vi "WHD_VEten_0.1_Pruebas.vi"() -> ()   [LabVIEW 2015]
uses:
  <vilib>/NI_Real-Time Target Support.lvlib
  <vilib>/rvi/interface/nirviReadWriteControl/nirviReadWriteControl.xnode
  <vilib>/rvi/interface/nirviMethod/nirviMethod.xnode
  <vilib>/rvi/interface/nirviOpenFPGA/nirviOpenFPGA.xnode
  <vilib>/rvi/interface/nirviCloseFPGA/nirviCloseFPGA.xnode
  <vilib>/real-time/NI_Real-Time Libraries.lvlib
  <vilib>/userdefined/High Color/nirio_resource_hc.ctl
  <vilib>/Utility/file.llb/Write To Spreadsheet File (string).vi
  AURA_Wheel/Json2Labv.lvlib
  AURA_Wheel/AuraWheelAPI/AuraWheel.lvlib
  <vilib>/LabVIEW Targets/FPGA/cRIO/shared/nicrio_ModuleControls/nicrio_cRIO-9234_DataRatesRing2.ctl
  FPGA Bitfiles/W&RDEuskotren_FPGATarget_FPGA8aws2_55B1237B.lvbitx
  <vilib>/real-time/rtutility.llb/RT Restart Target (Self).vi
  <vilib>/FPGAPlugInAG/cRIO-9113/niLvFpga_Open_cRIO-9113.vi
  <vilib>/FPGAPlugInAG/cRIO-9113/niLvFpga_Run_cRIO-9113.vi
  NiFpgaLv.dll
  <vilib>/Utility/error.llb/Error Cluster From Error Code.vi
  <vilib>/rvi/errors/niLvFpgaAdjustHostInterfaceError.vi
  <vilib>/FPGAPlugInAG/cRIO-9113/niLvFpga_ConfigureFifo_cRIO-9113.vi
  <vilib>/rvi/errors/niLvFpgaMergeErrorWithErrorCode.vi
  <vilib>/FPGAPlugInAG/cRIO-9113/niLvFpga_StartFifo_cRIO-9113.vi
  <vilib>/FPGAPlugInAG/cRIO-9113/niLvFpga_ReadFifo_cRIO-9113.vi
  <vilib>/FPGAPlugInAG/cRIO-9113/niLvFpga_StopFifo_cRIO-9113.vi
  <vilib>/FPGAPlugInAG/cRIO-9113/niLvFpga_Reset_cRIO-9113.vi
  <vilib>/FPGAPlugInAG/cRIO-9113/niLvFpga_Close_cRIO-9113.vi
  <vilib>/Utility/file.llb/Write Delimited Spreadsheet (string).vi
  <vilib>/RTwatchdog.llb/Watchdog expiration actions.ctl
panel:
  out "TAGs_AURAwheel":string[][](array[string])
  out "Plataformas?":bool
  out "Ejes_convoy":i32
  out "Nº Ejes":i32[](array[numeric])
  out "Nº UTs":i32
  out "it-read-LR6":i32[](array[numeric])
  out "it-LR6":i32
  out "RFID_LR6_Error":errorcluster
  out "TAGs HEX":string[](array[string])
  out "TAGs LR6":string[](array[string])
  in  "TAGs HEX 2":string[](array[string])
  out "Series_flota":string[](array[string])
  out "Tabla_flota":string[][](array[string])
  out "Puntos medios de las ventanas":dbl[][](array[numeric])
  in  "User":string
  in  "Índice de los archivos seleccionados":i32
  in  "Array":path[][](array[path])=[[path "c:/Trenes_prueba/0207_2013-09-24_19-09-42_0.bin", path "c:/Trenes_prueba/0096_2013-10-30_18-13-14_0.bin", path "c:/Trenes_prueba/0001_2013-06-05_13-06-23_0.bin"], [path "c:/Trenes_prueba/0207_2013-09-24_19-09-42_1.bin", path "c:/Trenes_prueba/0096_2013-10-30_18-13-14_1.bin", path "c:/Trenes_prueba/0001_2013-06-05_13-06-23_1.bin"], [path "c:/Trenes_prueba/0207_2013-09-24_19-09-42_2.bin", path "c:/Trenes_prueba/0096_2013-10-30_18-13-14_2.bin", path "c:/Trenes_prueba/0001_2013-06-05_13-06-23_2.bin"], [path "c:/Trenes_prueba/0207_2013-09-24_19-09-42_3.bin", path "c:/Trenes_prueba/0096_2013-10-30_18-13-14_3.bin", path "c:/Trenes_prueba/0001_2013-06-05_13-06-23_3.bin"], [path "c:/Trenes_prueba/0207_2013-09-24_19-09-42_4.bin", path "c:/Trenes_prueba/0096_2013-10-30_18-13-14_4.bin", path "c:/Trenes_prueba/0001_2013-06-05_13-06-23_4.bin"], [path "c:/Trenes_prueba/0207_2013-09-24_19-09-42_5.bin", path "c:/Trenes_prueba/0096_2013-10-30_18-13-14_5.bin", path "c:/Trenes_prueba/0001_2013-06-05_13-06-23_5.bin"], [path "c:/Trenes_prueba/0207_2013-09-24_19-09-42_6.bin", path "c:/Trenes_prueba/0096_2013-10-30_18-13-14_6.bin", path "c:/Trenes_prueba/0001_2013-06-05_13-06-23_6.bin"], [path "c:/Trenes_prueba/0207_2013-09-24_19-09-42_7.bin", path "c:/Trenes_prueba/0096_2013-10-30_18-13-14_7.bin", path "c:/Trenes_prueba/0001_2013-06-05_13-06-23_7.bin"], [path "c:/Trenes_prueba/0207_2013-09-24_19-09-42_8.bin", path "c:/Trenes_prueba/0096_2013-10-30_18-13-14_8.bin", path "c:/Trenes_prueba/0001_2013-06-05_13-06-23_8.bin"]]
  out "configuration file path":path=path "c:/Parametros.cfg"
  in  "IP synchr":string
  in  "Canal ccero?":bool
  in  "Digital?":bool=TRUE
  out "Numeric 3":i32
  out "data":cluster{"status":string}
  out "confRFID":path=path "c:/RFID/TAGS.csv"
  out "TAGS leidos":path=path "c:/RFID/TAGS.csv"
  in  "Use Aura?":bool
  in  "Parametros AuraWheel":string[](array[string])
  in  "Parámetros acelerómetros":dbl[](array[numeric])
  in  "Number of Samples":u32=2000
  in  "x*y":dbl[](array[numeric])=array[252000 elements]
  out "RFID_Error 2":errorcluster
  in  "milliseconds to wait":u32=180000
  in  "Adquirir continuado":bool
  in  "Tiempo de adquisicion":dbl=10.0
  in  "Adquirir":bool
  in  "Señal digital?":bool=TRUE
  out "Inductivo OK?":bool=TRUE
  out "Acelerómetros OK?":bool[](array[boolean])
  out "Fin":bool
  out "Contador":i32=1
  in  "expiration actions":T1={"reset"=TRUE, "occurrence"=FALSE, "trigger protocol"=enum."active high", "trigger line"=enum."none", "disable watchdog on VI exit"=TRUE}
  out "Path TEST":path=path "c:/TEST"
  out "Fallo fotocelula":bool
  out "Path_Borrar":path=path "c:/Trenes"
  out "Longitud de la unidad":dbl
  out "Bucle Espera":i32
  out "Aviso no detección":string
  out "Time to Acquire Block (ms)":i32
  out "Distancia de acelerómetros":dbl[](array[numeric])
  out "Block Size":u32
  out "Distancias generales":dbl[](array[numeric])
  in  "Reset del controlador":bool
  in  "Configuración":bool
  in  "Parar la aplicación":bool
  out "Acel 4":bool=TRUE
  out "Acel 3":bool=TRUE
  out "Acel 2":bool=TRUE
  out "Acel 1":bool=TRUE
  out "RFID":bool=TRUE
  out "date/time string":string
  out "Obstruido?":bool
  out "Tiempo":dbl
  out "Inicio pasada":timestamp
  out "Ultimo TEST":timestamp
  out "Fuente":bool=TRUE
  out "Estado":string
  in  "Number of Channels":u32=9
  out "RFID_ID":refnum<k5>
  out "DC OK":string
  out "Aviso temperatura":string
  in  "Tab Control":T2(tab)=enum."Parámetros"
  out "V (m/s)":dbl
  out "Temperatura (ºC)":dbl
  out "Max RMS Ruedas":dbl[][](array[numeric])
  in  "Hora de borrado":string
  out "result":bool
  out "TAGs":string[](array[string])
  out "Nombre de archivo":path[](array[path])
  out "Tiempo de paso (s)":dbl
  out "Tiempo extra de adquisición (s)":dbl
  out "Número de ejes detectados":i32
  out "Buffer Underflow":bool
  out "Buffer Overflow":bool
  out "Disco Duro Disponible (bytes)":i64
  out "created path":path
  out "Fallo sensores":string
  out "T fuera rango":bool
  in  "Frecuencia de muestreo (Hz)":dbl=25600.0
  in  "Escaneos de la FIFO por canal":u32=1000
  in  "Tiempo extra al detector de paso (s)":dbl=1.0
  in  "Filtro digital (ms)":u16=13
  in  "dt RMS":dbl=256.0
  in  "Time":T3 {"Segundo" min=0 max=60; "Minuto" min=0 max=60; "Hora" min=0 max=24}
  in  "Cambiar hora":bool
  in  "Date":T4={"Mes   "=1, "Día         "=1, "Año "=2010} {"Año" min=1900 max=3000 step=1; "Día" min=1 max=31 step=1; "Mes" min=1 max=12 step=1}
  in  "Cambiar Fecha":bool
  in  "Frecuencia de muestreo y módulo CRIO":T5=2 items=["51.200 kS/s (NI 9234)"=1, "25.600 kS/s (NI 9234)"=2, "17.067 kS/s (NI 9234)"=3, "12.800 kS/s (NI 9234)"=4, "10.240 kS/s (NI 9234)"=5, "8.533 kS/s (NI 9234)"=6, "7.314 kS/s (NI 9234)"=7, "6.400 kS/s (NI 9234)"=8, "5.689 kS/s (NI 9234)"=9, "5.120 kS/s (NI 9234)"=10, "4.654 kS/s (NI 9234)"=11, "4.267 kS/s (NI 9234)"=12, "3.938 kS/s (NI 9234)"=13, "3.657 kS/s (NI 9234)"=14, "3.413 kS/s (NI 9234)"=15, "3.200 kS/s (NI 9234)"=16, "3.012 kS/s (NI 9234)"=17, "2.845 kS/s (NI 9234)"=18, "2.695 kS/s (NI 9234)"=19, "2.560 kS/s (NI 9234)"=20, "2.438 kS/s (NI 9234)"=21, "2.328 kS/s (NI 9234)"=22, "2.226 kS/s (NI 9234)"=23, "2.133 kS/s (NI 9234)"=24, "2.048 kS/s (NI 9234)"=25, "1.969 kS/s (NI 9234)"=26, "1.896 kS/s (NI 9234)"=27, "1.829 kS/s (NI 9234)"=28, "1.765 kS/s (NI 9234)"=29, "1.707 kS/s (NI 9234)"=30, "1.652 kS/s (NI 9234)"=31]
  in  "Puerto RFID":u16=2189
  in  "IP RFID":string="192.168.106.99"
  in  "Offset_rueda":fxp<+/-,24,-4>=0.004999998956918716 format="%.27g"
  in  "Count(mSec)":u32=2
  in  "LR6 IP address":string="192.168.106.94"
  in  "Port LR6":u16=2001
  in  "Pruebas RFID 2":bool
  in  "Pruebas RFID 1":bool
  in  "Descargar":bool
  out "Parámetros":bool=TRUE
  out "Distacias y medidas de dispositivos":bool=TRUE
  out "RFID_Error":errorcluster
  out "error FPGA":errorcluster
  out "error manipulacion archivos":errorcluster
  out "Unidades y ejes":bool=TRUE
  out "RFID":bool=TRUE
  out "error AURA":errorcluster
  out "Response headers":string
  # "Funciona?"
  # "Inductivo"
  # "A4"
  # "A3"
  # "A1"
  # "A2"
  # "WRD_MEX\nWRD_ZAR"
  # "0 tagMexInit\n1 tagMexFin\n\n0 tag1\n1 tag2"
  # "Última detección de unidad"
  # "Error!!"
  # "Estado de la memoria"
  # "Espera"
  # "Adquisicion"
  # "Adquisicion"
  # "Procesado"
  # "Procesado"
  # "Procesado"
  # "Procesado"
  # "Procesado"
  # "Parámetros de muestreo"
  # "Parámetros de adquisición"
  # "Parámetros de procesado"
  # "Cambio Fecha y Hora"
  # "Descarga de planos y TEST"
  # "NO"
  # "SI"
  # "Descarga archivos binarios de adquisición"
  # "NO"
  # "SI"
  # "Cargar datos de configuración"
  # "Errores!!"
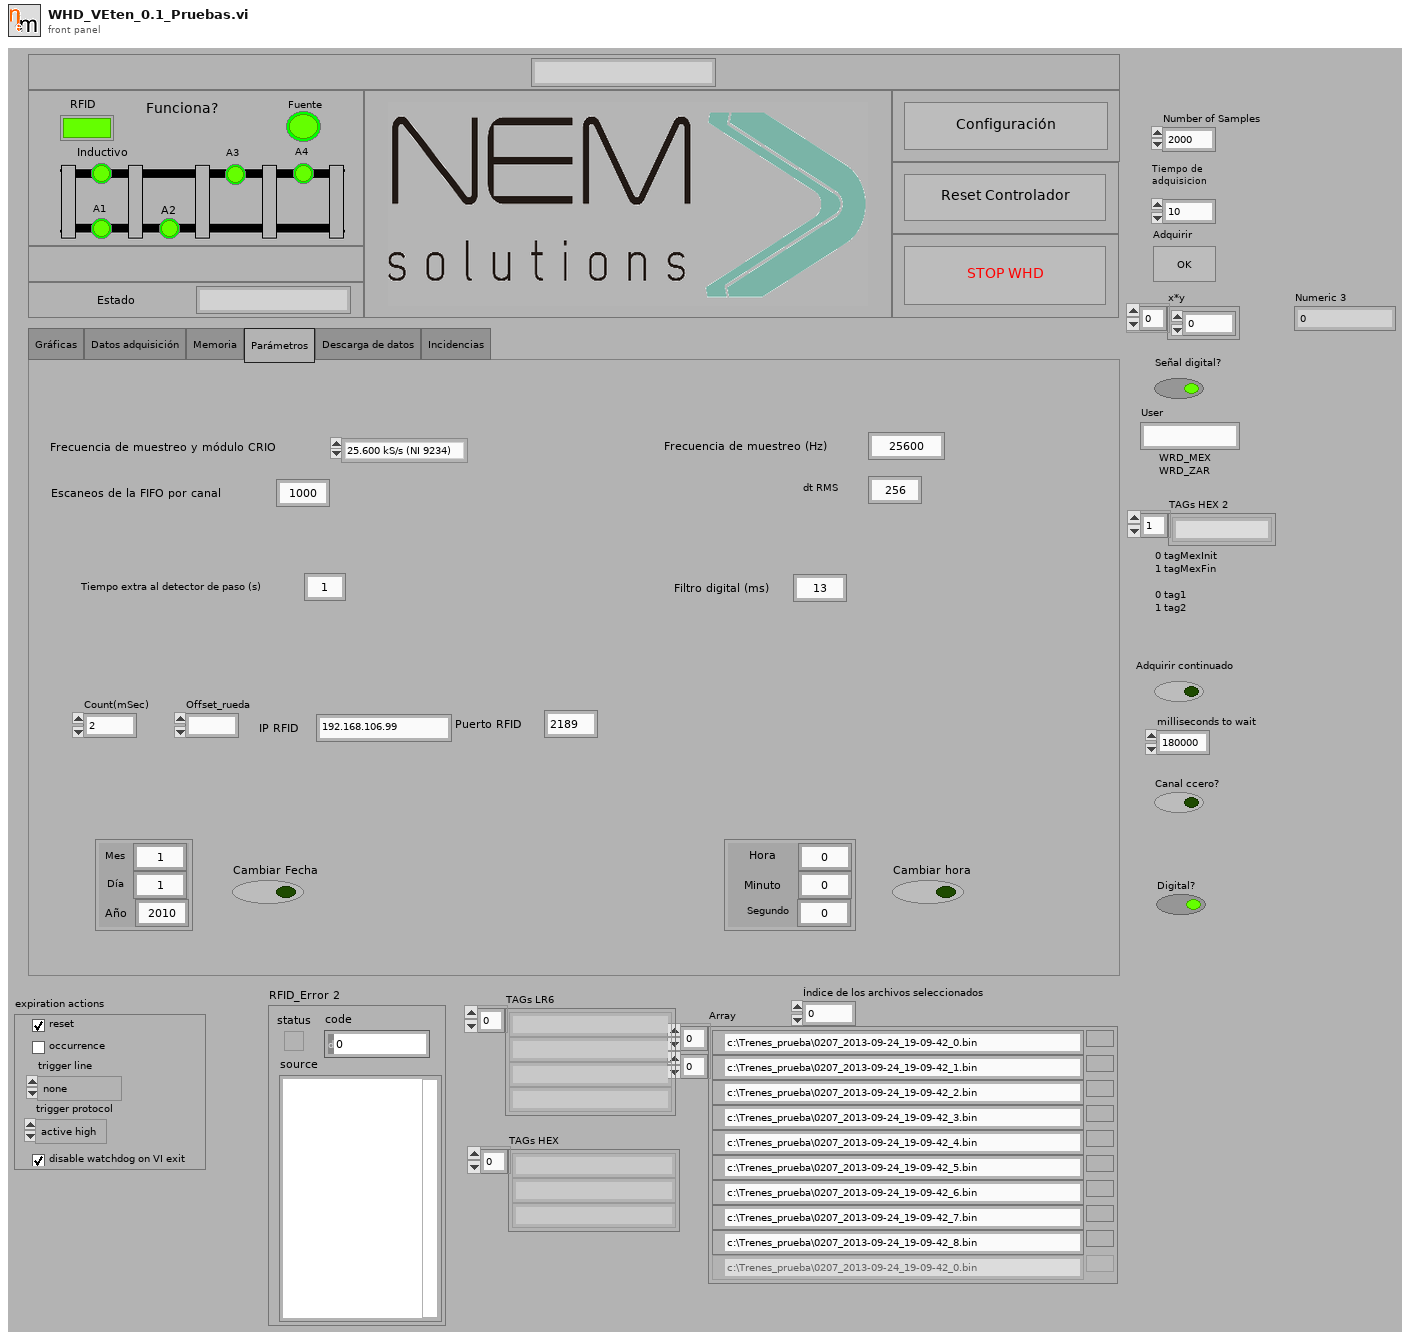
[diagram p1: front panel]
types:
  T1 = typedef "Watchdog expiration actions.ctl" = cluster{"reset":bool, "occurrence":bool, "trigger protocol":enum16{"active high", "active low", "open collector"}, "trigger line":enum16{"none", "line 0", "line 1", "line 2", "line 3", "line 4", "line 5", "line 6", "line 7", "SMB line 0"}, "disable watchdog on VI exit":bool}
  T2 = enum32{"Gráficas", "Datos adquisición", "Memoria", "Parámetros", "Descarga de datos", "Incidencias"}
  T3 = cluster{"Hora        ":i32, "Minuto     ":i32, "Segundo               ":i32}
  T4 = cluster{"Mes   ":i32, "Día         ":i32, "Año ":i32}
  T5 = typedef "nicrio_cRIO-9234_DataRatesRing2.ctl" = u8
  T6 = typedef "nirio_resource_hc.ctl" = tag
  T7 = enum16{"Standard", "Buffered", "CRLF", "Immediate"}
  T8 = enum16{"open", "replace", "create", "open or create", "replace or create", "replace or create with confirmation"}
  T9 = enum16{"big-endian, network order", "native, host order", "little-endian"}
  T10 = cluster{"error IO":errorcluster, bool[], u32[], string[], dbl[]}
  T11 = cluster{"g_ts":dbl, "p_sp":dbl, "p_tp":dbl, "p_tg":cluster{"tg_n":dbl, "tg_t":string}[], "p_ax":cluster{"ax_n":dbl, "ax_sp":dbl, "ax_wh":cluster{"wh_p":dbl, "wh_a1":dbl, "wh_a2":dbl, "wh_a3":dbl, "wh_a4":dbl}[]}[]}
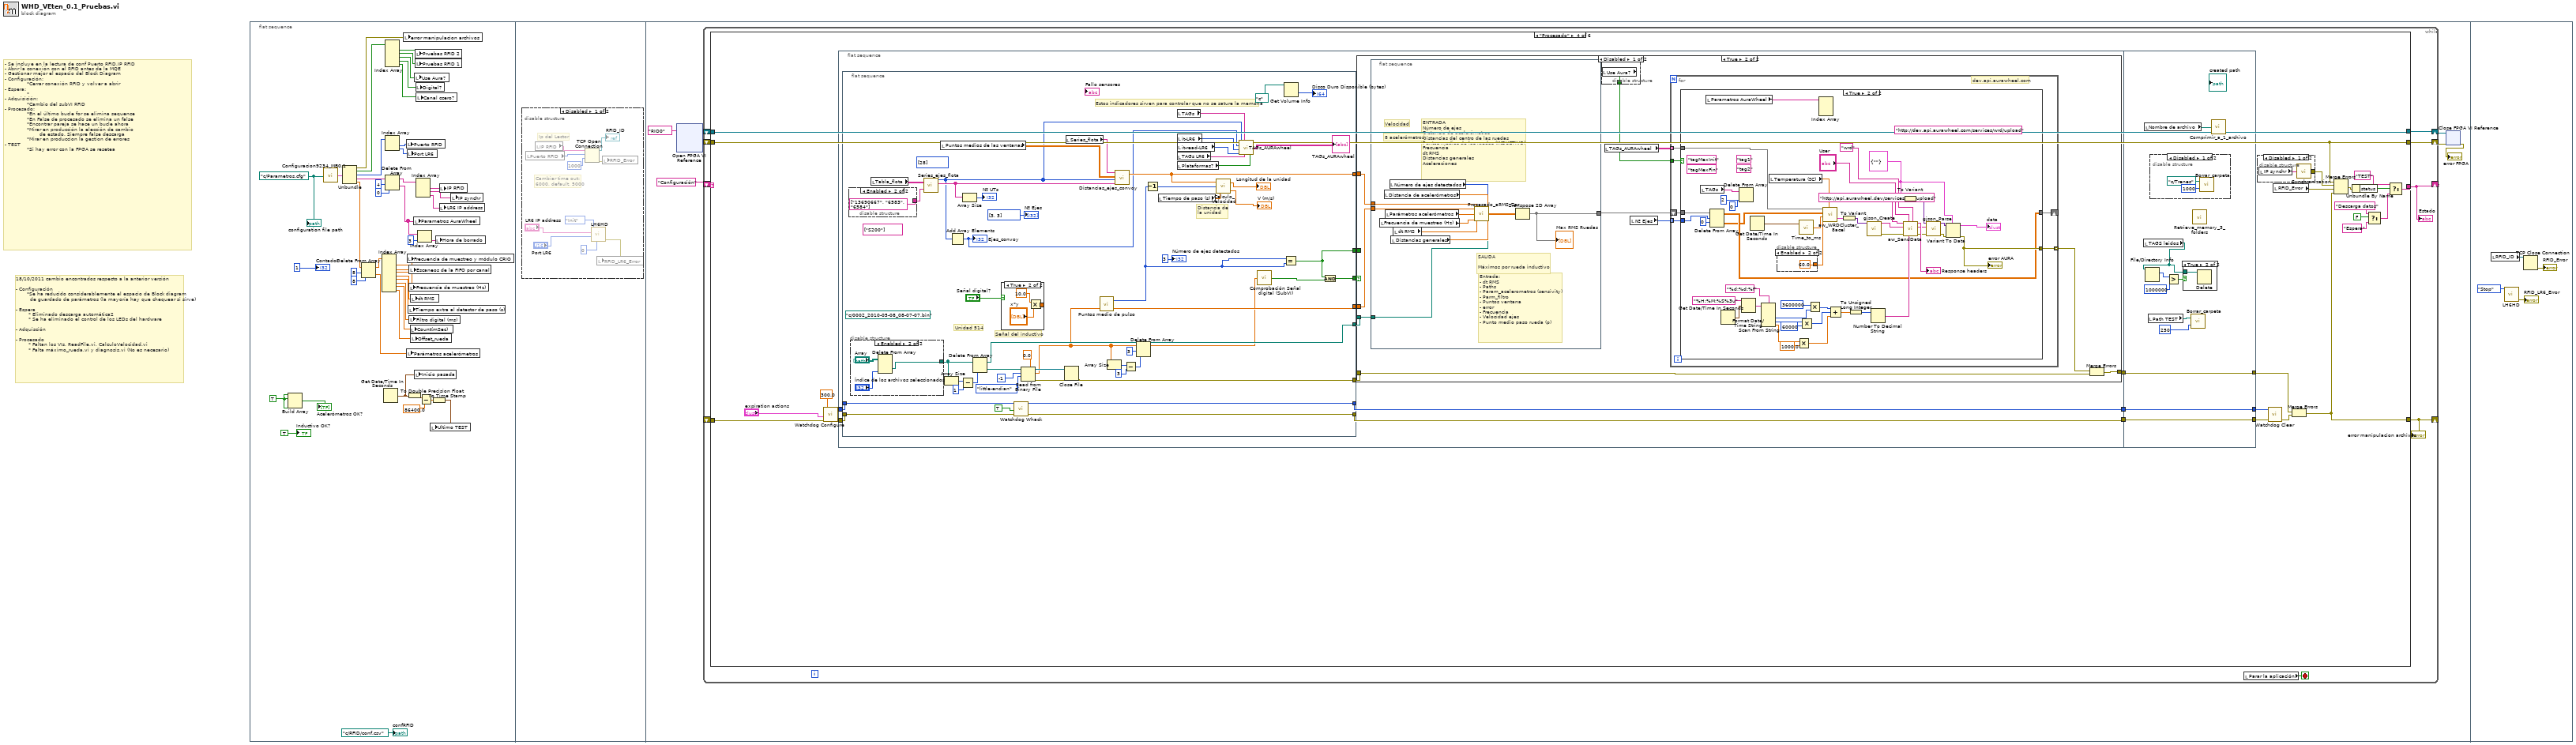
[diagram p0: block diagram]
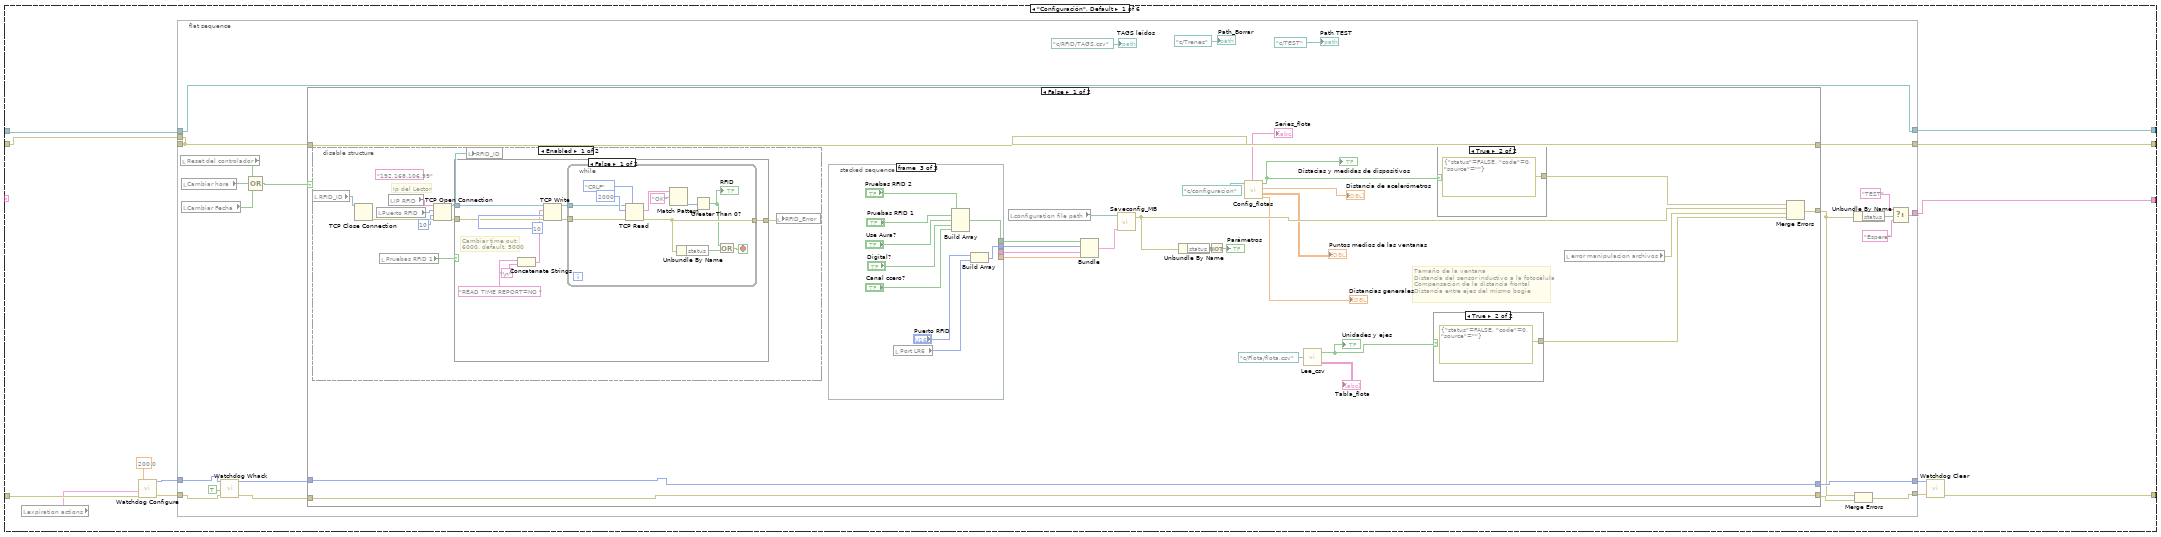
[diagram p3: hidden frame]
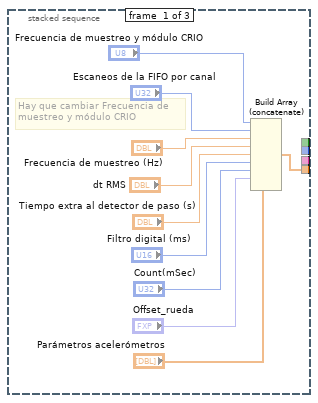
[diagram p4: hidden frame]
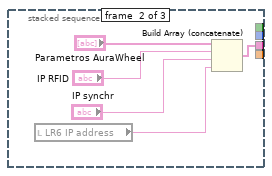
[diagram p5: hidden frame]
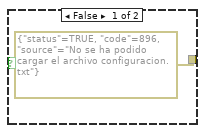
[diagram p6: hidden frame]
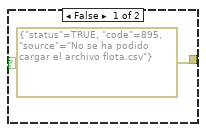
[diagram p7: hidden frame]
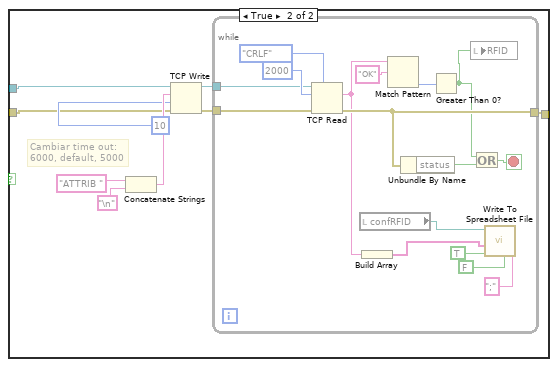
[diagram p8: hidden frame]
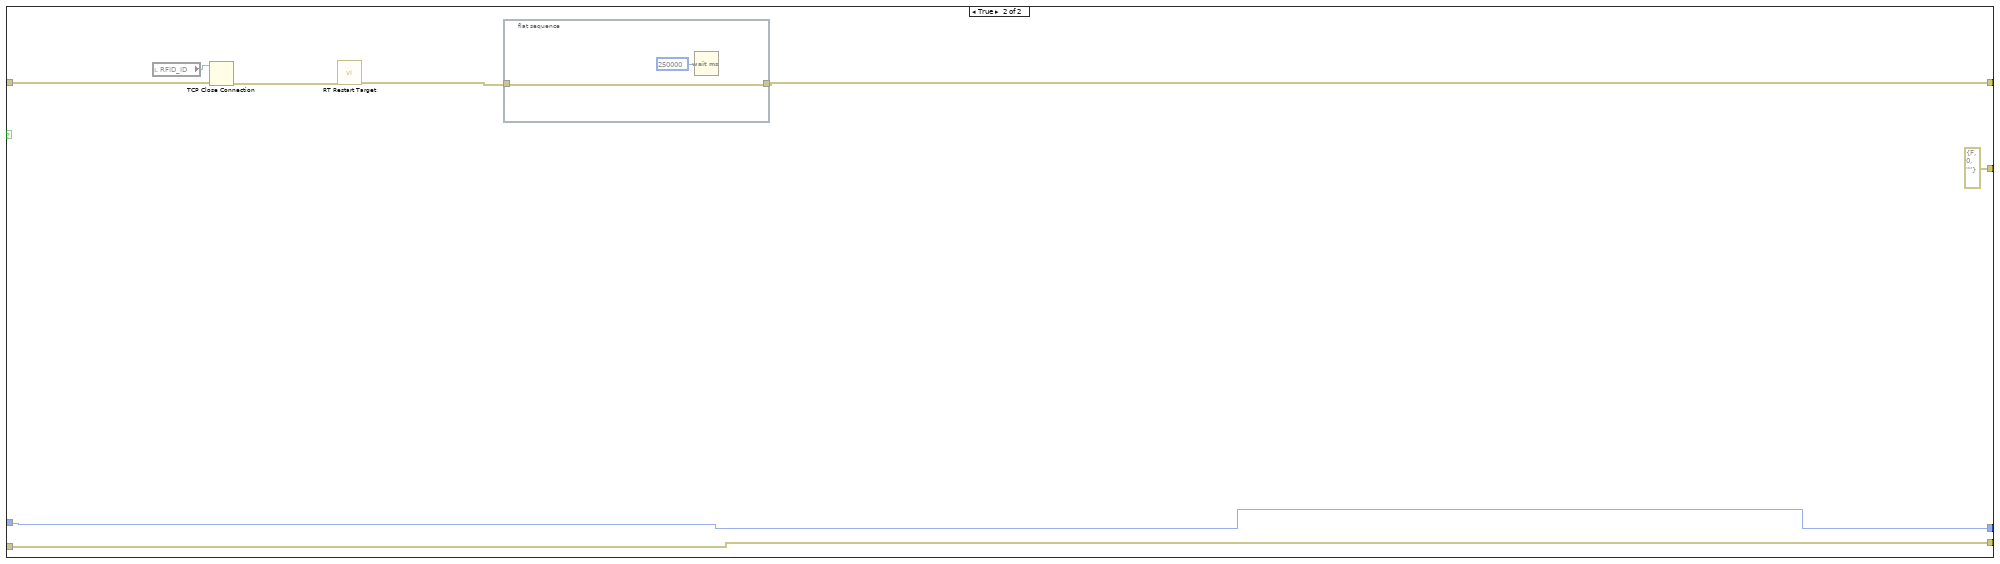
[diagram p10: hidden frame]
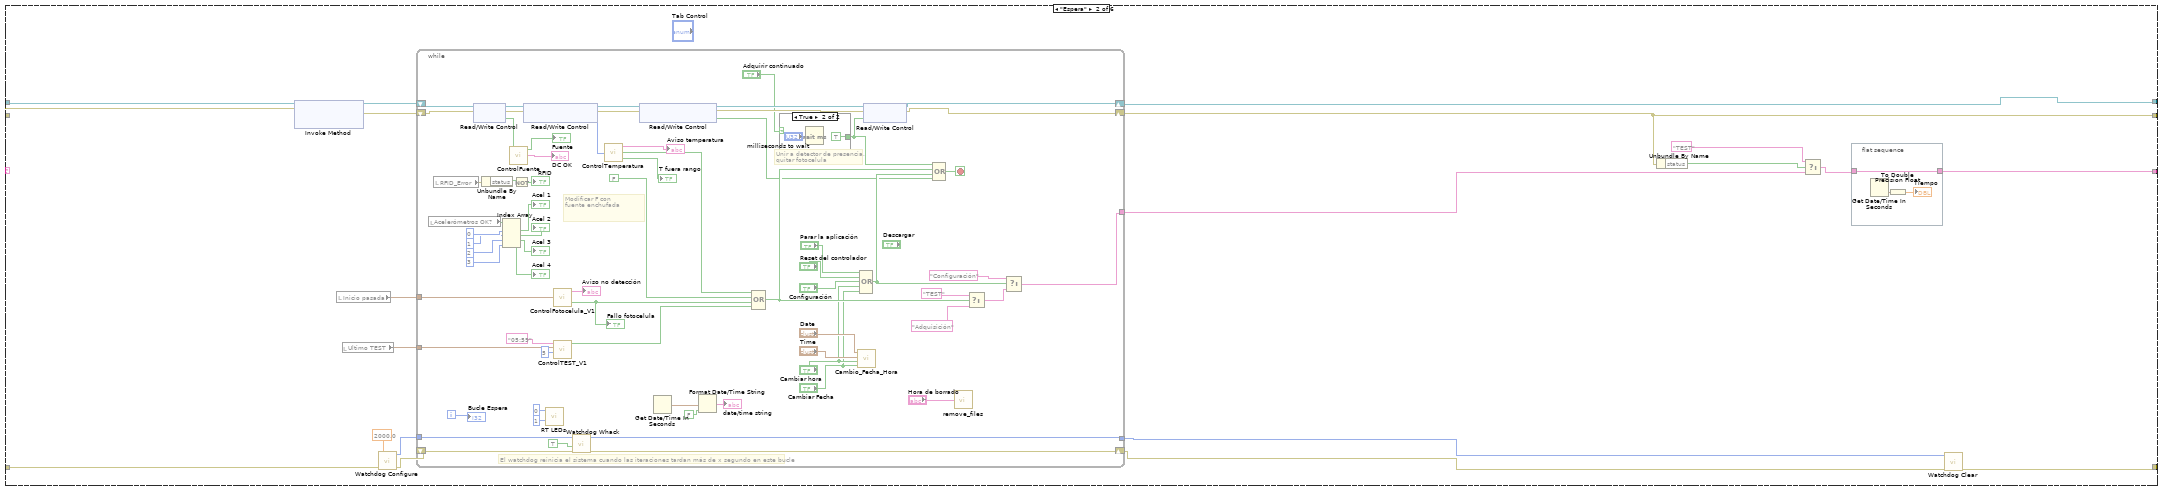
[diagram p11: hidden frame]
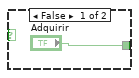
[diagram p12: hidden frame]
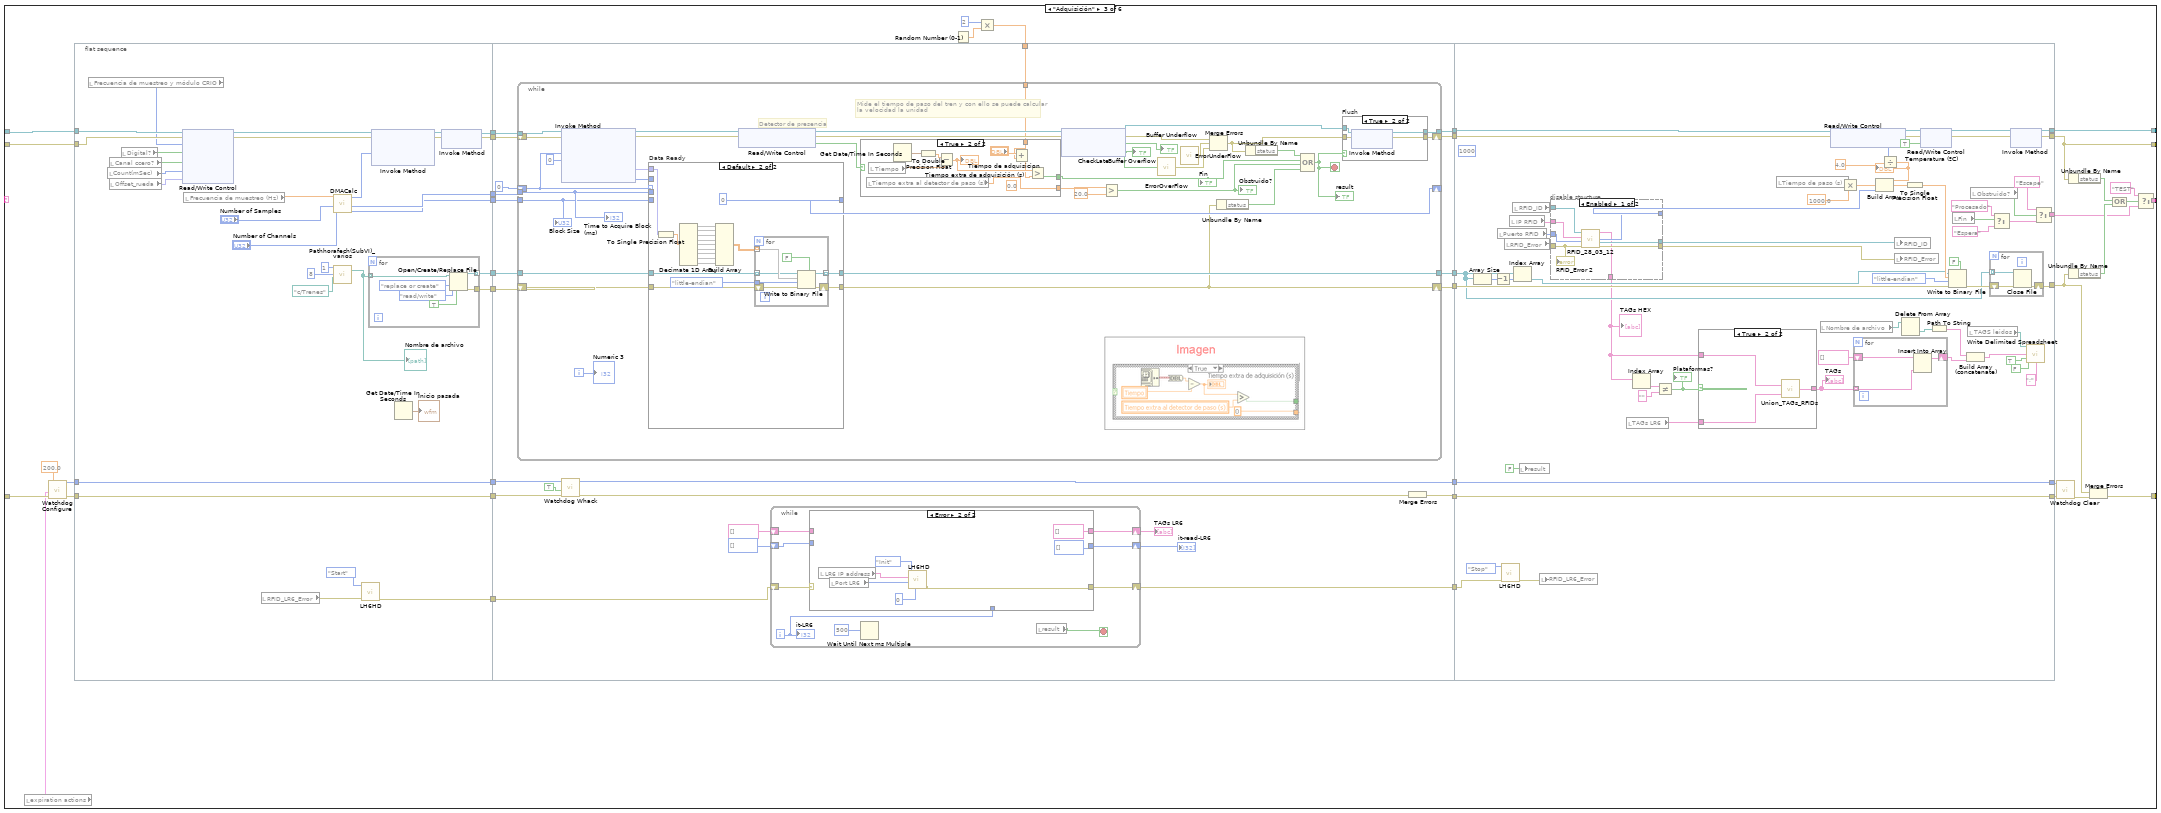
[diagram p13: hidden frame]
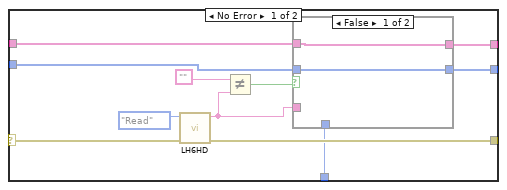
[diagram p14: hidden frame]
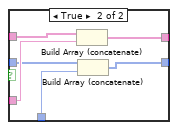
[diagram p15: hidden frame]
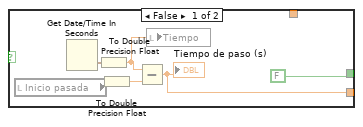
[diagram p16: hidden frame]
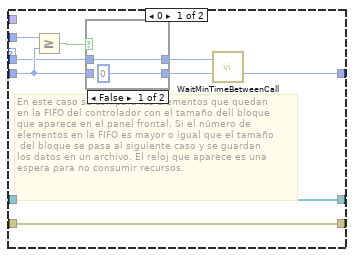
[diagram p17: hidden frame]
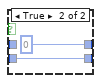
[diagram p18: hidden frame]
diagram:
  # "18/10/2011 cambio encontrados respecto a la anterior versión\n\n- Configuración\n       *Se ha reducido considerablemente el espacio de Block diagram\n         de guardado de parámetros (la mayoría hay que chequear si sirve)\n\n- Espera\n        * Eliminado descarga automática2\n        * Se ha eliminado el control de los LEDs del hardware\n       \n- Adquisción\n\n- Procesado\n        * Faltan los VIs, ReadFile.vi, CalculoVelocidad.vi\n        * Falta máximo_rueda.vi y diagnosis.vi (No es necesario)"
  # "- Se incluye en la lectura de conf Puerto RFID,IP RFID\n- Abrir la conexión con el RFID antes de la MQE\n- Gestionar mejor el espacio del Block Diagram\n- Configuración:\n              *Cerrar conexión RFID y volver a abrir\n- Espera:\n              *\n- Adquisición:\n              *Cambio del subVI RFID\n- Procesado:\n              *En el último bucle for se elimina sequence\n              *En False de procesado se elimina un false\n              *Encontrar pareja se hace un bucle ahora\n              *Mirar en producción la elección de cambio\n                      de estado. Siempre false descarga \n              *Mirar en produccion la gestion de errores\n- TEST\n              *Si hay error con la FPGA se resetea"
  n1 = flat-sequence {
    frame #0 {
      w29 = TRUE
      w25 = path "c:/Parametros.cfg" ("configuration file path")
      n2 = Build Array(w29, w29, w29, w29) -> (→"Acelerómetros OK?":bool[])
      n3 = call "Configuracion9234_MB0.1.vi"("configuration file path"=w25) -> ("output cluster"=w24:T10)
      n4 = Unbundle(w24) -> ("error IO"=w32:errorcluster, w31:bool[], w30:u32[], w16:string[], w22:dbl[])
      n5 = Delete From Array(array=w22, length=8, index=8) -> (deleted portion=w18:dbl[], array with subset deleted=w21:dbl[])
      n6 = Index Array(array=w21) -> (element #1=w40:dbl, element #2=w39:dbl, element #3=w38:dbl, element #4=w37:dbl, element #5=w36:dbl, element #6=w35:dbl, element #7=w8:dbl, element #8=w7:dbl)  [unwired: 8 in]
      n7 = Get Date/Time In Seconds() -> (seconds since 1Jan1904=w42:timestamp)
      n8 = Index Array(array=w31) -> (element #1=w34:bool, element #2=w33:bool, element #3=w17:bool, element #4=w4:bool, element #5=w9:bool)  [unwired: 5 in]
      n9 = Index Array(array=w30) -> (element #1=w23:u32, element #2=w1:u32)  [unwired: 2 in]
      n10 = Delete From Array(array=w16, length=4, index=0) -> (deleted portion=w5:string[], array with subset deleted=w15:string[])
      n11 = local write "error manipulacion archivos"(w32) -> ()
      n12 = local write "Puerto RFID"(w23) -> ()
      n13 = local write "Parámetros acelerómetros"(w18) -> ()
      n14 = local write "Port LR6"(w1) -> ()
      n15 = local write "Frecuencia de muestreo y módulo CRIO"(w40) -> ()
      n16 = To Double Precision Float(number=w42) -> (double precision float=w44:dbl)
      n17 = local write "Tiempo extra al detector de paso (s)"(w36) -> ()
      n18 = local write "Frecuencia de muestreo (Hz)"(w38) -> ()
      n19 = local write "Filtro digital (ms)"(w35) -> ()
      n20 = local write "Escaneos de la FIFO por canal"(w39) -> ()
      n21 = local write "Count(mSec)"(w8) -> ()
      n22 = local write "dt RMS"(w37) -> ()
      n23 = local write "Offset_rueda"(w7) -> ()
      n24 = local write "Parametros AuraWheel"(w5) -> ()
      n25 = local write "Inicio pasada"(w42) -> ()
      n26 = local write "Use Aura?"(w17) -> ()
      n27 = local write "Pruebas RFID 2"(w34) -> ()
      n28 = local write "Pruebas RFID 1"(w33) -> ()
      n29 = local write "Digital?"(w4) -> ()
      n30 = Index Array(array=w15) -> (element #1=w3:string, element #2=w6:string, element #3=w2:string)  [unwired: 3 in]
      n31 = local write "Canal ccero?"(w9) -> ()
      n32 = Index Array(array=w5, index=3) -> (element=w10:string)
      n33 = Subtract(x=w44, y=86400.0) -> (x-y=w43:dbl)
      n34 = To Time Stamp(1:w43) -> (0:w41:timestamp)
      n35 = local write "Ultimo TEST"(w41) -> ()
      n36 = local write "Hora de borrado"(w10) -> ()
      n37 = local write "IP RFID"(w3) -> ()
      n38 = local write "LR6 IP address"(w2) -> ()
      n39 = local write "IP synchr"(w6) -> ()
      "Contador" <- 1
      "Inductivo OK?" <- TRUE ("Inductivo OK?")
      "confRFID" <- path "c:/RFID/conf.csv" ("file path (use dialog)")
      "configuration file path" <- w25
    }
    frame #1 {
      n40 = disable-structure shown="Disabled" {
        frame Disabled {
          # "Cambiar time out:\n6000, default, 5000"
          # "Ip del Lector"
          n41 = local read "Puerto RFID"() -> (w52:u16)
          n42 = local read "IP RFID"() -> (w53:string)
          n43 = TCP Open Connection(address=w53, remote port or service name=w52, timeout ms (60000)=1000) -> (connection ID=→"RFID_ID":refnum<k5>, error out=w51:errorcluster)  [unwired: 1 in, 1 out]
          n44 = call "LH6HD.vi"("DeviceAddress"=u8 0, "Reader Port"="Port LR6", "IP Address"="LR6 IP address", "Action"=enum16{"Init", "Start", "Read", "Stop", "Exit"}."Init") -> ("error out"=w50:errorcluster)  [unwired: 6 in, 1 out]
          n45 = local write "RFID_LR6_Error"(w50) -> ()
          n46 = local write "RFID_Error"(w51) -> ()
        }
        frame Enabled {
        }
      }
    }
    frame #2 {
      n47 = xnode "Open FPGA VI Reference"("resource name"=T6 "RIO0") -> ("FPGA VI Reference Out"=w62:refnum<k20>, "error out"=w61:errorcluster)  [unwired: 1 in]
      n48 = while {
        shift-right: [w66] -> _
        shift-left: "Configuración" -> [w71]
        shift-right: [w64] -> w58
        shift-left: w62 -> [w70]
        shift-right: [w63] -> w57
        shift-left: w61 -> [w69]
        shift-right: [w68] -> _
        shift-left: _ -> [w67]
        stop <- w65 stop-if-true
        n49 = case shown="\"Procesado\"" w71 {
          tunnel: [w83 w228 w324 w638 w858 "TEST" ("t")] -> w66
          tunnel: [w82 w227 w345 w653 w856 w925] -> w64
          tunnel: [w84 w225 w346 w630 w847 w922] -> w63
          tunnel: w70 -> [w73 w234 w356 w653 w856 w924]
          tunnel: w69 -> [w72 w232 w355 w630 w855 w921]
          tunnel: [w75 w226 w341 w635 w854 w926] -> w68
          tunnel: w67 -> [w80 w242 w347 w651 w857 w926]
          frame "Configuración", Default {
            n50 = local read "expiration actions"() -> (w74:T1)
            n51 = call <vilib>:"Watchdog Configure.vi"("error in (no error)"=w80, "expiration actions"=w74, "timeout (1 sec)"=200.0) -> ("error out"=w79:errorcluster, "watchdogID"=w78:u64)  [unwired: 3 out]
            n52 = flat-sequence {
              tunnel: [w85] -> _
              tunnel: [w94] -> w84
              tunnel: [w106] -> w83
              tunnel: w73 -> [w95]
              tunnel: [w95] -> w82
              tunnel: w79 -> [w89]
              tunnel: w78 -> [w87]
              tunnel: [w93] -> w77
              tunnel: [w97] -> w76
              tunnel: w72 -> [w85]
              frame #0 {
                n53 = local read "Reset del controlador"() -> (w102:bool)
                n54 = local read "Cambiar hora"() -> (w101:bool)
                n55 = local read "Cambiar Fecha"() -> (w100:bool)
                n56 = call <vilib>:"Watchdog Whack.vi"("error in (no error)"=w89, "reset watchdog after expire? (F)"=TRUE, "watchdogID in"=w87) -> ("error out"=w88:errorcluster, "watchdogID out"=w86:u64)  [unwired: 3 out]
                n57 = Compound Arithmetic op=OR(w102, w101, w100) -> (w99:bool)
                n58 = case shown="False" w99 {
                  tunnel: w85 -> [w132 w220]
                  tunnel: [w132 w217] -> w94
                  tunnel: [w118 errorcluster {"status"=FALSE, "code"=0, "source"=""} ("error IO")] -> w92
                  tunnel: w86 -> [w117 w216]
                  tunnel: w88 -> [w116 w215]
                  tunnel: [w117 w216] -> w93
                  tunnel: [w116 w215] -> w91
                  frame False {
                    # "Tamaño de la ventana\nDistancia del sensor inductivo a la fotocélula\nCompensación de la distancia frontal\nDistancia entre ejes del mismo bogie"
                    n59 = disable-structure shown="Enabled" {
                      frame Enabled {
                        (unwired) "192.168.106.99" ("address")
                        # "Ip del Lector"
                        n60 = local read "RFID_ID"() -> (w168:refnum<k5>)
                        n61 = TCP Close Connection(connection ID=w168) -> (error out=w169:errorcluster)  [unwired: 2 in, 1 out]
                        n62 = local read "Puerto RFID"() -> (w166:u16)
                        n63 = local read "Pruebas RFID 1"() -> (w161:bool)
                        n64 = local read "IP RFID"() -> (w165:string)
                        n65 = TCP Open Connection(address=w165, remote port or service name=w166, timeout ms (60000)=10, error in (no error)=w169) -> (connection ID=w167:refnum<k5>, error out=w162:errorcluster)  [unwired: 1 out]
                        n66 = case shown="False" w161 {
                          tunnel: w167 -> [w178 w192]
                          tunnel: [w176 w190] -> w163
                          tunnel: w162 -> [w173 w191]
                          frame False {
                            # "Cambiar time out:\n6000, default, 5000"
                            n67 = Concatenate Strings("READ TIME REPORT=NO " ("data in"), "\n") -> (w170:string)
                            n68 = TCP Write(connection ID=w178, data in=w170, error in (no error)=w173, 9:10 ("timeout ms (25000)")) -> (connection ID out=w174:refnum<k5>, error out=w175:errorcluster)  [unwired: 1 out]
                            n69 = while {
                              tunnel: w175 -> [w187]
                              tunnel: w174 -> [w186]
                              tunnel: [w185] -> w176
                              stop <- w182 stop-if-true
                              n70 = TCP Read(connection ID=w186, bytes to read=2000, error in (no error)=w187, 7:T7."CRLF" ("mode (standard)")) -> (data out=w180:string, error out=w185:errorcluster)  [unwired: 1 in, 1 out]
                              n71 = Match Pattern(string=w180, regular expression="OK") -> (offset past match=w183:i32)  [unwired: 4 out]
                              n72 = Unbundle By Name(w185) -> ("status"=w181:bool)
                              n73 = Greater Than 0?(x=w183) -> (x > 0?=w179:bool)
                              "RFID" <- w179
                              n74 = Or(x=w179, y=w181) -> (x .or. y?=w182:bool)
                            }
                          }
                          frame True {
                            # "Cambiar time out:\n6000, default, 5000"
                            n75 = Concatenate Strings("ATTRIB " ("data in"), "\n") -> (w198:string)
                            n76 = TCP Write(connection ID=w192, data in=w198, error in (no error)=w191, 9:10 ("timeout ms (25000)")) -> (connection ID out=w195:refnum<k5>, error out=w194:errorcluster)  [unwired: 1 out]
                            n77 = while {
                              tunnel: w194 -> [w212]
                              tunnel: w195 -> [w211]
                              tunnel: [w210] -> w190
                              stop <- w207 stop-if-true
                              n78 = TCP Read(connection ID=w211, bytes to read=2000, error in (no error)=w212, 7:T7."CRLF" ("mode (standard)")) -> (data out=w201:string, error out=w210:errorcluster)  [unwired: 1 in, 1 out]
                              n79 = local read "confRFID"() -> (w199:path)
                              n80 = Build Array(w201) -> (w200:string[])
                              n81 = Match Pattern(string=w201, regular expression="OK") -> (offset past match=w208:i32)  [unwired: 4 out]
                              n82 = Unbundle By Name(w210) -> ("status"=w206:bool)
                              n83 = Greater Than 0?(x=w208) -> (x > 0?=w205:bool)
                              n84 = local write "RFID"(w205) -> ()
                              n85 = Or(x=w205, y=w206) -> (x .or. y?=w207:bool)
                              n86 = call-poly <vilib>:"Write To Spreadsheet File.vi"("delimiter (\\t)"=";" ("delimiter (\\t)"), "transpose? (no:F)"=FALSE, "append to file? (new file:F)"=TRUE, "1D data"=w200, "file path (dialog if empty)"=w199) -> ()  [unwired: 3 in, 1 out]
                            }
                          }
                        }
                        n87 = local write "RFID_ID"(w167) -> ()
                        n88 = local write "RFID_Error"(w163) -> ()
                      }
                      frame Disabled {
                      }
                    }
                    n89 = stacked-sequence {
                      tunnel: [w137 _ _] -> w122
                      tunnel: [_ w147 _] -> w121
                      tunnel: [_ _ w153] -> w123
                      tunnel: [_ _ w152] -> w124
                      frame #0 {
                        # "Hay que cambiar Frecuencia de\nmuestreo y módulo CRIO"
                        n90 = Build Array (concatenate)("Frecuencia de muestreo y módulo CRIO", "Escaneos de la FIFO por canal", "Frecuencia de muestreo (Hz)", "dt RMS", "Tiempo extra al detector de paso (s)", "Filtro digital (ms)", "Count(mSec)", "Offset_rueda", "Parámetros acelerómetros") -> (w137:dbl[])
                      }
                      frame #1 {
                        n91 = local read "LR6 IP address"() -> (w143:string)
                        n92 = Build Array (concatenate)("Parametros AuraWheel", "IP RFID", "IP synchr", w143) -> (w147:string[])
                      }
                      frame #2 {
                        n93 = local read "Port LR6"() -> (w148:u16)
                        n94 = Build Array("Pruebas RFID 2", "Pruebas RFID 1", "Use Aura?", "Digital?", "Canal ccero?") -> (w152:bool[])
                        n95 = Build Array("Puerto RFID", w148) -> (w153:u16[])
                      }
                    }
                    n96 = local read "configuration file path"() -> (w119:path)
                    n97 = Bundle(w124, w123, w121, w122) -> (w120:cluster{bool[], u16[], string[], dbl[]})  [unwired: 1 in]
                    n98 = call "Saveconfig_MB.vi"("configuration file path"=w119, "Configuracion"=w120) -> ("error out"=w127:errorcluster)  [unwired: 4 in]
                    n99 = Unbundle By Name(w127) -> ("status"=w128:bool)
                    n100 = Not(x=w128) -> (.not. x?=→"Parámetros":bool)
                    n101 = call "Config_flotas.vi"("file path (dialog if empty)"=path "c:/configuracion") -> ("Distancias generales"=→"Distancias generales":dbl[], "Puntos medios de las ventanas"=→"Puntos medios de las ventanas":dbl[][], "Distancia de acelerómetros"=→"Distancia de acelerómetros":dbl[], "Distacias y medidas de dispositivos"=w115:bool, "Series_flota"=→"Series_flota":string[])  [unwired: 3 in]
                    "Distacias y medidas de dispositivos" <- w115
                    n102 = call "Lee_csv.vi"("Path"=path "c:/Flota/flota.csv") -> ("Tabla_flota"=→"Tabla_flota":string[][], "Lectura_OK?"=w111:bool)
                    "Unidades y ejes" <- w111
                    n103 = case shown="True" w111 {
                      tunnel: [errorcluster {"status"=TRUE, "code"=895, "source"="No se ha podido cargar el archivo flota.csv"} ("error out") errorcluster {"status"=FALSE, "code"=0, "source"=""} ("error out")] -> w125
                      frame False {
                      }
                      frame True {
                      }
                    }
                    n104 = case shown="True" w115 {
                      tunnel: [errorcluster {"status"=TRUE, "code"=896, "source"="No se ha podido cargar el archivo configuracion.txt"} ("error out") errorcluster {"status"=FALSE, "code"=0, "source"=""} ("error out")] -> w130
                      frame False {
                      }
                      frame True {
                      }
                    }
                    n105 = local read "error manipulacion archivos"() -> (w126:errorcluster)
                    n106 = Merge Errors(w130, w127, w126, w125) -> (w118:errorcluster)
                  }
                  frame True {
                    n107 = local read "RFID_ID"() -> (w222:refnum<k5>)
                    n108 = TCP Close Connection(connection ID=w222, error in (no error)=w220) -> (error out=w219:errorcluster)  [unwired: 2 out]
                    n109 = call-poly <vilib>:"RT Restart Target.vi"("error in (no error)"=w219) -> ("error out"=w218:errorcluster)  [unwired: 10 in]
                    n110 = flat-sequence {
                      tunnel: [w224] -> w217
                      tunnel: w218 -> [w224]
                      frame #0 {
                        n111 = Wait (ms)(milliseconds to wait=u32 250000) -> ()  [unwired: 1 out]
                      }
                    }
                  }
                }
                n112 = Unbundle By Name(w92) -> ("status"=w107:bool)
                n113 = Merge Errors(w92, w91) -> (w97:errorcluster)
                n114 = Select(t="TEST", s=w107, f="Espera") -> (s? t:f=w106:string)
                "Path_Borrar" <- path "c:/Trenes" ("file path (use dialog)")
                "Path TEST" <- path "c:/TEST" ("file path (use dialog)")
                "TAGS leidos" <- path "c:/RFID/TAGS.csv" ("file path (use dialog)")
              }
            }
            n115 = call <vilib>:"Watchdog Clear.vi"("error in (no error)"=w76, "watchdogID in"=w77) -> ("error out"=w75:errorcluster)  [unwired: 5 out]
          }
          frame "Espera" {
            n116 = xnode "Invoke Method"("FPGA VI Reference In"=w234, "error in"=w232) -> ("FPGA VI Reference Out"=w233:refnum<k20>, "error out"=w231:errorcluster)  [unwired: 1 in]
            n117 = local read "Inicio pasada"() -> (w239:timestamp)
            n118 = local read "Ultimo TEST"() -> (w238:timestamp)
            n119 = call <vilib>:"Watchdog Configure.vi"("error in (no error)"=w242, "timeout (1 sec)"=2000.0) -> ("error out"=w243:errorcluster, "watchdogID"=w244:u64)  [unwired: 1 in, 3 out]
            n120 = while {
              tunnel: [w264] -> w237
              tunnel: w244 -> [w312]
              tunnel: [w310] -> w241
              shift-right: [w250] -> w227
              shift-left: w233 -> [w266]
              shift-right: [w251] -> w225
              shift-left: w231 -> [w265]
              tunnel: w239 -> [w277]
              tunnel: w238 -> [w276]
              shift-right: [w275] -> w230
              shift-left: w243 -> [w311]
              i -> [w303]
              stop <- w314 stop-if-true
              # "Modificar F con\nfuente enchufada"
              # "Unir a detector de presencia,\nquitar fotocelula"
              # "El watchdog reinicia el sistema cuando las iteraciones tardan más de x segundo en este bucle"
              n121 = local read "Acelerómetros OK?"() -> (w274:bool[])
              n122 = local read "RFID_Error"() -> (w286:errorcluster)
              n123 = xnode "Read/Write Control"("FPGA VI Reference In"=w266, "error in"=w265) -> ("FPGA VI Reference Out"=w298:refnum<k20>, "error out"=w297:errorcluster, "DC OK"=w302:bool)
              n124 = Unbundle By Name(w286) -> ("status"=w284:bool)
              n125 = Index Array(array=w274, index #1=0 ("index"), index #2=1 ("index"), index #3=2 ("index"), index #4=3 ("index")) -> (element #1=→"Acel 1":bool, element #2=→"Acel 2":bool, element #3=→"Acel 3":bool, element #4=→"Acel 4":bool)
              n126 = call "ControlFuente.vi"("DC OK 3"=w302) -> ("DC OK 2"=→"Fuente":bool, "DC OK"=→"DC OK":string)  [unwired: 1 out]
              n127 = Not(x=w284) -> (.not. x?=→"RFID":bool)
              n128 = xnode "Read/Write Control"("FPGA VI Reference In"=w298, "error in"=w297) -> ("FPGA VI Reference Out"=w293:refnum<k20>, "error out"=w292:errorcluster, "Chassis Temperature"=w300:i16)
              n129 = call <vilib>:"RT LEDs.vi"("State"=1, "LED Num"=0) -> ()  [unwired: 1 in, 5 out]
              n130 = call "ControlFotocelula_V1.vi"("Tiempo de entrada a espera"=w277) -> ("Aviso no detección"=→"Aviso no detección":string, "Boolean"=w290:bool)
              "Fallo fotocelula" <- w290
              n131 = call "ControlTEST_V1.vi"("Días entre TEST 2"=i16 5, "Ultimo TEST"=w276, "Horario TEST"="05:59") -> ("Boolean"=w289:bool)  [unwired: 3 in]
              n132 = call <vilib>:"Watchdog Whack.vi"("error in (no error)"=w311, "reset watchdog after expire? (F)"=TRUE, "watchdogID in"=w312) -> ("error out"=w275:errorcluster, "watchdogID out"=w310:u64)  [unwired: 3 out]
              n133 = call "ControlTemperatura.vi"("Chassis Temperature"=w300) -> ("Aviso temperatura"=→"Aviso temperatura":string, "Boolean"=w294:bool, "T fuera rango"=→"T fuera rango":bool)
              n134 = xnode "Read/Write Control"("FPGA VI Reference In"=w293, "error in"=w292) -> ("FPGA VI Reference Out"=w269:refnum<k20>, "error out"=w268:errorcluster, "Detector de presencia"=w254:bool)
              n135 = Get Date/Time In Seconds() -> (seconds since 1Jan1904=w256:timestamp)
              n136 = Format Date/Time String(seconds (now)=w256, UTC format=FALSE) -> (date/time string=→"date/time string":string)  [unwired: 1 in]
              n137 = Compound Arithmetic op=OR(w294, FALSE ("value"), w290, w289) -> (w291:bool)
              n138 = case shown="True" "Adquirir continuado" {
                tunnel: ["Adquirir" TRUE ("Adquirir")] -> w263
                frame False {
                }
                frame True {
                  n139 = Wait (ms)(milliseconds to wait="milliseconds to wait") -> ()  [unwired: 1 out]
                }
              }
              n140 = call "Cambio_Fecha_Hora.vi"("Cambiar Fecha"="Cambiar Fecha", "Cambiar hora"="Cambiar hora", "Time"="Time", "Date"="Date") -> ()
              n141 = Compound Arithmetic op=OR("Parar la aplicación", "Reset del controlador", "Configuración", "Cambiar hora", "Cambiar Fecha") -> (w287:bool)
              n142 = xnode "Read/Write Control"("FPGA VI Reference In"=w269, "error in"=w268, "Fotocélula"=w263) -> ("FPGA VI Reference Out"=w250:refnum<k20>, "error out"=w251:errorcluster)
              n143 = Compound Arithmetic op=OR(w263, w291, w287, w254) -> (w314:bool)
              n144 = call "remove_files.vi"("Hora de borrado"="Hora de borrado") -> ()  [unwired: 1 in]
              n145 = Select(t="TEST", s=w291, f="Adquisición") -> (s? t:f=w306:string)
              n146 = Select(t="Configuración", s=w287, f=w306) -> (s? t:f=w264:string)
              "Bucle Espera" <- w303
            }
            n147 = Unbundle By Name(w225) -> ("status"=w236:bool)
            n148 = Select(t="TEST", s=w236, f=w237) -> (s? t:f=w229:string)
            n149 = flat-sequence {
              tunnel: [w246] -> w228
              tunnel: w229 -> [w246]
              frame #0 {
                n150 = Get Date/Time In Seconds() -> (seconds since 1Jan1904=w247:timestamp)
                n151 = To Double Precision Float(number=w247) -> (double precision float=→"Tiempo":dbl)
              }
            }
            n152 = call <vilib>:"Watchdog Clear.vi"("error in (no error)"=w230, "watchdogID in"=w241) -> ("error out"=w226:errorcluster)  [unwired: 5 out]
          }
          frame "Adquisición" {
            n153 = local read "expiration actions"() -> (w323:T1)
            n154 = call <vilib>:"Watchdog Configure.vi"("error in (no error)"=w347, "expiration actions"=w323, "timeout (1 sec)"=200.0) -> ("error out"=w331:errorcluster, "watchdogID"=w332:u64)  [unwired: 3 out]
            n155 = flat-sequence {
              tunnel: w331 -> [w386]
              tunnel: w332 -> [w387]
              tunnel: w355 -> [w380]
              tunnel: w356 -> [w381]
              tunnel: [w387] -> w340
              tunnel: [w386] -> w339
              tunnel: [w379] -> w338
              tunnel: [w378] -> w337
              tunnel: [w377] -> w336
              tunnel: [w376] -> w335
              tunnel: [w375] -> w334
              tunnel: [w374] -> w333
              tunnel: [w357] -> w319
              tunnel: [w416] -> w353
              tunnel: [w400] -> w352
              tunnel: [w415] -> w351
              tunnel: [w414] -> w350
              tunnel: [w411] -> w349
              tunnel: [w404] -> w348
              tunnel: w340 -> [w413]
              tunnel: w339 -> [w412]
              tunnel: w338 -> [w410]
              tunnel: w337 -> [w409]
              tunnel: w336 -> [w408]
              tunnel: w335 -> [w407]
              tunnel: w334 -> [w406]
              tunnel: w333 -> [w405]
              tunnel: w320 -> [w403]
              tunnel: w319 -> [w398]
              tunnel: [w397] -> w318
              tunnel: w353 -> [w589]
              tunnel: w352 -> [w588]
              tunnel: w351 -> [w573]
              tunnel: w350 -> [w572]
              tunnel: w349 -> [w561]
              tunnel: [w596] -> w327
              tunnel: w348 -> [w599]
              tunnel: [w579] -> w342
              tunnel: [w580] -> w346
              tunnel: [w581] -> w345
              tunnel: [w589] -> w344
              tunnel: [w588] -> w343
              tunnel: w318 -> [w554]
              frame #0 {
                n156 = local read "Frecuencia de muestreo y módulo CRIO"() -> (w364:T5)
                n157 = local read "Count(mSec)"() -> (w361:u32)
                n158 = local read "Canal ccero?"() -> (w362:bool)
                n159 = local read "Offset_rueda"() -> (w360:fxp<+/-,24,-4>)
                n160 = local read "Digital?"() -> (w363:bool)
                n161 = xnode "Read/Write Control"("FPGA VI Reference In"=w381, "error in"=w380, "Data Rate"=w364, "Digital?"=w363, "Canal ccero?"=w362, "Count(mSec)"=w361, "Offset_rueda"=w360) -> ("FPGA VI Reference Out"=w370:refnum<k20>, "error out"=w369:errorcluster)
                n162 = local read "Frecuencia de muestreo (Hz)"() -> (w372:dbl)
                n163 = local read "RFID_LR6_Error"() -> (w358:errorcluster)
                n164 = call "DMACalc.vi"("Number of Channels"="Number of Channels", "Number of Samples"="Number of Samples", "Rate (Hz)"=w372) -> ("Block Size"=w376:u32, "Time to Acquire Block (ms)"=w377:i32, "Host Buffer Size"=w382:u32)  [unwired: 6 in]
                n165 = call "Pathhorafech(SubVI)_varios.vi"("Folder path"=path "c:/Trenes", "Nº de acelerómetros"=8, "Nº inductivos"=1) -> ("Acel_Paths"=w365:path[])  [unwired: 1 in, 1 out]
                "Nombre de archivo" <- w365
                n166 = call "LH6HD.vi"("error in (no error)"=w358, "Action"=enum16{"Init", "Start", "Read", "Stop", "Exit"}."Start") -> ("error out"=w357:errorcluster)  [unwired: 8 in, 1 out]
                n167 = for {
                  tunnel: w365 -> [w390] mode=indexing
                  tunnel: [w389] -> w375 mode=indexing
                  tunnel: [w388] -> w374
                  n168 = Open/Create/Replace File(file path (use dialog)=w390, operation (0:open)=T8."replace or create", access (0:read/write)=enum16{"read/write", "read-only", "write-only"}."read/write", disable buffering (F)=TRUE) -> (refnum out=w389:refnum<file>, error out=w388:errorcluster)  [unwired: 1 in, 2 out]
                }
                n169 = xnode "Invoke Method"("FPGA VI Reference In"=w370, "error in"=w369, "Requested Depth"=w382) -> ("FPGA VI Reference Out"=w385:refnum<k20>, "error out"=w384:errorcluster)  [unwired: 1 out]
                n170 = Get Date/Time In Seconds() -> (seconds since 1Jan1904=→"Inicio pasada":timestamp)
                n171 = xnode "Invoke Method"("FPGA VI Reference In"=w385, "error in"=w384) -> ("FPGA VI Reference Out"=w379:refnum<k20>, "error out"=w378:errorcluster)
              }
              frame #1 {
                n172 = while "Data Acquisition" {
                  tunnel: w410 -> [w457]
                  shift-right: [w486] -> _
                  shift-left: u32 0 ("t") -> [w482]
                  tunnel: w408 -> [w487]
                  tunnel: w407 -> [w485]
                  shift-right: [w488] -> w414
                  shift-left: w409 -> [w479]
                  tunnel: [w483] -> w415
                  tunnel: w406 -> [w463]
                  tunnel: [w464] -> w411
                  shift-right: [w462] -> w404
                  shift-left: w405 -> [w475]
                  tunnel: w403 -> [w459]
                  i -> [w456]
                  stop <- w484 stop-if-true
                  # "Detector de presencia"
                  # "Mide el tiempo de paso del tren y con ello se puede calcular\nla velocidad la unidad"
                  n173 = xnode "Invoke Method"("FPGA VI Reference In"=w457, "error in"=w479, "Number of Elements"=w482, "Timeout (ms)"=0) -> ("FPGA VI Reference Out"=w453:refnum<k20>, "error out"=w461:errorcluster, "Data"=w478:fxp<+/-,24,4>[], "Elements Remaining"=w480:u32)
                  n174 = case "Data Ready" shown="Default" w482 {
                    tunnel: w487 -> [w508 _]
                    tunnel: [w507 u32 0 ("t")] -> w486
                    tunnel: w485 -> [w509 _]
                    tunnel: w480 -> [w506 _]
                    tunnel: w478 -> [_ w530]
                    tunnel: w475 -> [w505 w529]
                    tunnel: [w505 w531] -> w462
                    tunnel: w463 -> [w504 w528]
                    tunnel: [w504 w527] -> w464
                    frame 0 {
                      # "En este caso se compara los elementos que quedan\nen la FIFO del controlador con el tamaño dell bloque\nque aparece en el panel frontal. Si el número de \nelementos en la FIFO es mayor o igual que el tamaño\n del bloque se pasa al siguiente caso y se guardan \nlos datos en un archivo. El reloj que aparece es una\nespera para no consumir recursos."
                      n175 = Greater Or Equal?(x=w506, y=w509) -> (x >= y?=w510:bool)
                      n176 = case shown="False" w510 {
                        tunnel: [u32 0 ("Block Size") w514] -> w507
                        tunnel: [w513 0 ("t")] -> w511
                        tunnel: w508 -> [w513 _]
                        tunnel: w509 -> [_ w514]
                        frame False {
                        }
                        frame True {
                        }
                      }
                      n177 = call "WaitMinTimeBetweenCall.vi"("Minimum ms between calls"=w511) -> ()  [unwired: 2 in]
                    }
                    frame Default {
                      n178 = To Single Precision Float(number=w530) -> (single precision float=w517:sgl[])
                      n179 = Decimate 1D Array(w517) -> (w523:sgl[], w526:sgl[], w525:sgl[], w524:sgl[], w522:sgl[], w521:sgl[], w520:sgl[], w519:sgl[], w518:sgl[])
                      n180 = Build Array(w523, w526, w525, w524, w522, w521, w520, w519, w518) -> (w516:sgl[][])
                      n181 = for {
                        tunnel: T9."little-endian" ("byte order (0:big-endian, network order)") -> [w540]
                        shift-right: [w534] -> w531
                        shift-left: w529 -> [w535]
                        tunnel: w516 -> [w538] mode=indexing
                        tunnel: w528 -> [w537] mode=indexing
                        tunnel: [w536] -> w527 mode=indexing
                        n182 = Write to Binary File(file (use dialog)=w537, data=w538, error in=w535, 5:FALSE ("prepend array or string size? (T)"), 9:w540) -> (refnum out=w536:refnum<file>, error out=w534:errorcluster)  [unwired: 2 out]
                      }
                    }
                  }
                  n183 = xnode "Read/Write Control"("FPGA VI Reference In"=w453, "error in"=w461) -> ("FPGA VI Reference Out"=w477:refnum<k20>, "error out"=w476:errorcluster, "Detector de presencia"=w469:bool)
                  n184 = case shown="True" w469 {
                    tunnel: [FALSE w499] -> w468
                    tunnel: [w490 w498] -> w467
                    tunnel: w459 -> [_ w495]
                    frame False {
                      n185 = local read "Inicio pasada"() -> (w493:timestamp)
                      n186 = Get Date/Time In Seconds() -> (seconds since 1Jan1904=w492:timestamp)
                      n187 = To Double Precision Float(number=w492) -> (double precision float=w489:dbl)
                      n188 = To Double Precision Float(number=w493) -> (double precision float=w494:dbl)
                      n189 = Subtract(x=w489, y=w494) -> (x-y=w490:dbl)
                      "Tiempo de paso (s)" <- w490
                      n190 = local write "Tiempo"(w489) -> ()
                    }
                    frame True {
                      (unwired) 0.0
                      n191 = local read "Tiempo extra al detector de paso (s)"() -> (w498:dbl)
                      n192 = local read "Tiempo"() -> (w503:dbl)
                      n193 = Get Date/Time In Seconds() -> (seconds since 1Jan1904=w500:timestamp)
                      n194 = To Double Precision Float(number=w500) -> (double precision float=w501:dbl)
                      n195 = Subtract(x=w501, y=w503) -> (x-y=w502:dbl)
                      "Tiempo extra de adquisición (s)" <- w502
                      n196 = Add(x="Tiempo de adquisicion", y=w495) -> (x+y=w496:dbl)
                      n197 = Greater?(x=w502, y=w496) -> (0:w499:bool)
                    }
                  }
                  "Fin" <- w468
                  n198 = xnode ("CheckLate")("FPGA VI Reference In"=w477, "error in"=w476) -> ("FPGA VI Reference Out"=w455:refnum<k20>, "error out"=w472:errorcluster, "Buffer Underflow"=→"Buffer Underflow":bool, "Buffer Overflow"=w458:bool)
                  "Buffer Overflow" <- w458
                  n199 = Greater?(x=w467, y=20.0) -> (0:w465:bool)
                  "Obstruido?" <- w465
                  n200 = call "ErrorOverFlow.vi"("Buffer Overflow"=w458) -> ("error out"=w470:errorcluster)
                  n201 = call "ErrorUnderFlow.vi"() -> ("error out"=w471:errorcluster)  [unwired: 1 in]
                  n202 = Merge Errors(w472, w471, w470) -> (w454:errorcluster)
                  n203 = Unbundle By Name(w462) -> ("status"=w466:bool)
                  n204 = Unbundle By Name(w454) -> ("status"=w474:bool)
                  n205 = Compound Arithmetic op=OR(w474, w468, w465, w466) -> (w484:bool)
                  "result" <- w484
                  n206 = case "Flush" shown="True" w484 {
                    tunnel: [w541 w546] -> w488
                    tunnel: [w542 w545] -> w483
                    tunnel: w455 -> [w542 w544]
                    tunnel: w454 -> [w541 w543]
                    frame False {
                    }
                    frame True {
                      n207 = xnode "Invoke Method"("FPGA VI Reference In"=w544, "error in"=w543) -> ("FPGA VI Reference Out"=w545:refnum<k20>, "error out"=w546:errorcluster)
                    }
                  }
                  "Block Size" <- w485
                  "Time to Acquire Block (ms)" <- w487
                  "Numeric 3" <- w456
                }
                n208 = call <vilib>:"Watchdog Whack.vi"("error in (no error)"=w412, "reset watchdog after expire? (F)"=TRUE, "watchdogID in"=w413) -> ("error out"=w401:errorcluster, "watchdogID out"=w416:u64)  [unwired: 3 out]
                n209 = while {
                  shift-right: [w424] -> w397
                  shift-left: w398 -> [w425]
                  shift-right: [w423] -> w396
                  shift-left: string[] [] -> [w422]
                  shift-right: [w418] -> w394
                  shift-left: i32[] [] -> [w419]
                  i -> [w420]
                  stop <- w421 stop-if-true
                  n210 = case shown="Error" w425 {
                    selector: w425 -> [w436 _]
                    tunnel: [w435 w450] -> w424
                    tunnel: [w431 string[] []] -> w423
                    tunnel: w422 -> [w430 _]
                    tunnel: w420 -> [w429 _]
                    tunnel: w419 -> [w428 _]
                    tunnel: [w427 i32[] []] -> w418
                    frame No Error {
                      n211 = call "LH6HD.vi"("error in (no error)"=w436, "Action"=enum16{"Init", "Start", "Read", "Stop", "Exit"}."Read") -> ("error out"=w435:errorcluster, "Tag"=w432:string)  [unwired: 8 in]
                      n212 = Not Equal?(x="", y=w432) -> (x != y?=w433:bool)
                      n213 = case shown="False" w433 {
                        tunnel: w432 -> [_ w445]
                        tunnel: [w439 w444] -> w431
                        tunnel: w430 -> [w439 w443]
                        tunnel: w429 -> [_ w440]
                        tunnel: w428 -> [w438 w442]
                        tunnel: [w438 w441] -> w427
                        frame False {
                        }
                        frame True {
                          n214 = Build Array (concatenate)(w443, w445) -> (w444:string[])
                          n215 = Build Array (concatenate)(w442, w440) -> (w441:i32[])
                        }
                      }
                    }
                    frame Error {
                      n216 = local read "LR6 IP address"() -> (w447:string)
                      n217 = local read "Port LR6"() -> (w448:u16)
                      n218 = call "LH6HD.vi"("DeviceAddress"=u8 0, "Reader Port"=w448, "IP Address"=w447, "Action"=enum16{"Init", "Start", "Read", "Stop", "Exit"}."Init") -> ("error out"=w450:errorcluster)  [unwired: 6 in, 1 out]
                    }
                  }
                  n219 = Wait Until Next ms Multiple(millisecond multiple=u32 500) -> ()  [unwired: 1 out]
                  n220 = local read "result"() -> (w421:bool)
                  "it-LR6" <- w420
                }
                "TAGs LR6" <- w396
                "it-read-LR6" <- w394
                n221 = Merge Errors(w401) -> (w400:errorcluster)
              }
              frame #2 {
                (unwired) u32 1000 ("Number of Elements")
                n222 = Array Size(array=w561) -> (size(s)=w559:i32)
                n223 = Decrement(x=w559) -> (x-1=w560:i32)
                n224 = local read "Puerto RFID"() -> (w578:u16)
                n225 = call "LH6HD.vi"("error in (no error)"=w554, "Action"=enum16{"Init", "Start", "Read", "Stop", "Exit"}."Stop") -> ("error out"=w553:errorcluster)  [unwired: 8 in, 1 out]
                n226 = local read "RFID_Error"() -> (w592:errorcluster)
                n227 = local read "IP RFID"() -> (w558:string)
                n228 = local read "RFID_ID"() -> (w591:refnum<k5>)
                n229 = Index Array(array=w561, index=w560) -> (element=w569:refnum<file>)
                n230 = local write "result"(FALSE ("result")) -> ()
                n231 = local write "RFID_LR6_Error"(w553) -> ()
                n232 = disable-structure shown="Enabled" {
                  disable-tunnel: [w623 _] -> w593
                  disable-tunnel: w592 -> [w622 w625]
                  disable-tunnel: w591 -> [w621 _]
                  disable-tunnel: [w620 _] -> w590
                  disable-tunnel: [w619 w625] -> w582
                  disable-tunnel: w578 -> [w618 _]
                  disable-tunnel: w558 -> [w617 _]
                  disable-tunnel: [w616 "TAGs HEX 2"] -> w551
                  frame Enabled {
                    n233 = call "RFID_28_03_12.vi"("RFID_Error"=w622, "Puerto RFID"=w618, "IP RFID"=w617, "RFID ID"=w621) -> ("Unidad"=w623:u32, "RFID Error"=w619:errorcluster, "connection ID out"=w620:refnum<k5>, "TAGs HEX"=w616:string[])  [unwired: 1 in]
                    "RFID_Error 2" <- w622
                  }
                  frame Disabled {
                  }
                }
                "TAGs HEX" <- w551
                n234 = local read "TAGs LR6"() -> (w552:string[])
                n235 = Index Array(array=w551) -> (element=w550:string)  [unwired: 1 in]
                n236 = Not Equal?(x=w550, y="" ("delimiter (\\t)")) -> (x != y?=w548:bool)
                "Plataformas?" <- w548
                n237 = case shown="True" w548 {
                  tunnel: w552 -> [w609 w610]
                  tunnel: [w609 w612] -> w556
                  tunnel: w551 -> [_ w611]
                  frame False {
                  }
                  frame True {
                    n238 = call "Union_TAGs_RFIDs.vi"("TAGs LR6"=w610, "TAGs HEX"=w611) -> ("TAGs"=w612:string[])
                  }
                }
                "TAGs" <- w556
                n239 = local read "Tiempo de paso (s)"() -> (w586:dbl)
                n240 = local read "Nombre de archivo"() -> (w568:path[])
                n241 = xnode "Read/Write Control"("FPGA VI Reference In"=w573, "error in"=w572) -> ("FPGA VI Reference Out"=w595:refnum<k20>, "error out"=w594:errorcluster, "Chassis Temperature"=w605:i16)
                n242 = Multiply(x=w586, y=1000.0) -> (x*y=w584:dbl)
                n243 = for {
                  shift-right: [w628] -> w576
                  shift-left: string[] [] -> [w627]
                  tunnel: w556 -> [w626] mode=indexing
                  n244 = Insert Into Array(array=w627, new element=w626) -> (w628:string[])  [unwired: 1 in]
                }
                n245 = Divide(x=w605, y=4.0) -> (x/y=w606:dbl)
                "Temperatura (ºC)" <- w606
                n246 = Build Array(w606, w584, w593) -> (w600:dbl[])
                n247 = local write "RFID_ID"(w590) -> ()
                n248 = local write "RFID_Error"(w582) -> ()
                n249 = Delete From Array(array=w568) -> (deleted portion=w567:path)  [unwired: 2 in, 1 out]
                n250 = To Single Precision Float(number=w600) -> (single precision float=w603:sgl[])
                n251 = xnode "Read/Write Control"("FPGA VI Reference In"=w595, "error in"=w594, "Stop"=TRUE ("stop")) -> ("FPGA VI Reference Out"=w571:refnum<k20>, "error out"=w570:errorcluster)
                n252 = Path To String(path=w567) -> (string=w575:string)
                n253 = Write to Binary File(file (use dialog)=w569, data=w603, error in=w599, 5:FALSE ("prepend array or string size? (T)"), 9:T9."little-endian" ("byte order (0:big-endian, network order)")) -> (error out=w566:errorcluster)  [unwired: 3 out]
                n254 = local read "Fin"() -> (w583:bool)
                n255 = Build Array (concatenate)(w575, w576) -> (w547:string[])
                n256 = local read "TAGS leidos"() -> (w562:path)
                n257 = local read "Obstruido?"() -> (w587:bool)
                n258 = for {
                  shift-right: [w615] -> w579
                  shift-left: w566 -> [w614]
                  tunnel: w561 -> [w613] mode=indexing
                  n259 = Close File(refnum=w613, error in=w614) -> (error out=w615:errorcluster)  [unwired: 1 out]
                }
                n260 = Select(t="Procesado", s=w583, f="Espera") -> (s? t:f=w598:string)
                n261 = xnode "Invoke Method"("FPGA VI Reference In"=w571, "error in"=w570) -> ("FPGA VI Reference Out"=w581:refnum<k20>, "error out"=w580:errorcluster)
                n262 = call-poly <vilib>:"Write Delimited Spreadsheet.vi"("file path (dialog if empty)"=w562, "1D data"=w547, "append to file? (F)"=FALSE ("transpose? (no:F)"), "transpose? (F)"=TRUE ("append to file? (new file:F)"), "delimiter (\\t)"=";" ("delimiter (\\t)")) -> ()  [unwired: 9 in, 2 out]
                n263 = Select(t="Escape", s=w587, f=w598) -> (s? t:f=w596:string)
              }
            }
            n264 = Random Number (0-1)() -> (number: 0 to 1=w322:dbl)
            n265 = Multiply(x=2, y=w322) -> (x*y=w320:dbl)
            n266 = call <vilib>:"Watchdog Clear.vi"("error in (no error)"=w343, "watchdogID in"=w344) -> ("error out"=w330:errorcluster)  [unwired: 5 out]
            n267 = Unbundle By Name(w346) -> ("status"=w328:bool)
            n268 = Unbundle By Name(w342) -> ("status"=w329:bool)
            n269 = Merge Errors(w342, w330) -> (w341:errorcluster)
            n270 = Compound Arithmetic op=OR(w328, w329) -> (w326:bool)
            n271 = Select(t="TEST", s=w326, f=w327) -> (s? t:f=w324:string)
          }
          frame "Procesado" {
            n272 = call <vilib>:"Watchdog Configure.vi"("error in (no error)"=w651, "expiration actions"="expiration actions", "timeout (1 sec)"=300.0) -> ("error out"=w649:errorcluster, "watchdogID"=w650:u64)  [unwired: 3 out]
            n273 = flat-sequence {
              tunnel: w650 -> [w663]
              tunnel: w649 -> [w662]
              tunnel: [w666] -> w633
              tunnel: [w661] -> w632
              tunnel: [w660] -> w631
              tunnel: [w841] -> w647
              tunnel: [w842] -> w648
              tunnel: [w843] -> w644
              tunnel: w633 -> [w843]
              tunnel: w632 -> [w842]
              tunnel: w631 -> [w841]
              frame #0 {
                n274 = flat-sequence {
                  tunnel: [w710] -> w665
                  tunnel: [w692] -> w664
                  tunnel: w663 -> [w717]
                  tunnel: w662 -> [w716]
                  tunnel: [w715] -> w661
                  tunnel: [w714] -> w660
                  tunnel: [w695] -> w659
                  tunnel: [w679] -> w658
                  tunnel: [w694] -> w657
                  tunnel: [w678] -> w656
                  frame #0 {
                    (unwired) string[] ["S200"] ("Series_flota1")
                    (unwired) i32[] [28] ("Ejes_UT")
                    (unwired) path "c:/0002_2010-05-08_08-07-07.bin" ("Nombre de archivo")
                    # "Unidad 514"
                    # "Señal del inductivo"
                    # "Estos indicadores sirven para controlar que no se sature la memoria"
                    # "Distancia de\nla unidad"
                    n275 = disable-structure shown="Enabled" {
                      disable-tunnel: [w719 string[] ["13690667", "6583", "6584"] ("Series_flota1")] -> w683
                      frame Disabled {
                        n276 = local read "TAGs"() -> (w719:string[])
                      }
                      frame Enabled {
                      }
                    }
                    n277 = disable-structure shown="Enabled" {
                      disable-tunnel: [w721 w723] -> w705
                      frame Disabled {
                        n278 = local read "Nombre de archivo"() -> (w721:path[])
                      }
                      frame Enabled {
                        n279 = Delete From Array(array="Array", index (col)="Índice de los archivos seleccionados") -> (deleted portion=w723:path[])  [unwired: 2 in, 1 out]
                      }
                    }
                    n280 = local read "Tabla_flota"() -> (w691:string[][])
                    n281 = call "Series_ejes_flota.vi"("Tabla_flota"=w691, "Tags"=w683) -> ("Nº Ejes"=w672:i32[], "Series del convoy"=w682:string[])  [unwired: 2 in, 1 out]
                    n282 = local read "Puntos medios de las ventanas"() -> (w693:dbl[][])
                    n283 = Array Size(array=w705) -> (size(s)=w702:i32)
                    n284 = Add Array Elements(numeric array=w672) -> (sum=w671:i32)
                    "Ejes_convoy" <- w671
                    n285 = Subtract(x=w702, y=1 ("length")) -> (x-y=w704:i32)
                    n286 = Array Size(array=w682) -> (size(s)=→"Nº UTs":i32)
                    n287 = Delete From Array(array=w705, index=w704) -> (deleted portion=w701:path, array with subset deleted=w694:path[])  [unwired: 1 in]
                    n288 = case shown="True" "Señal digital?" {
                      tunnel: [sgl[] [5.23] ("x*y") w728] -> _
                      frame False {
                      }
                      frame True {
                        n289 = Multiply(x=sgl 10.0, y="x*y") -> (x*y=w728:dbl[])
                      }
                    }
                    n290 = call <vilib>:"Watchdog Whack.vi"("error in (no error)"=w716, "reset watchdog after expire? (F)"=TRUE, "watchdogID in"=w717) -> ("error out"=w715:errorcluster, "watchdogID out"=w714:u64)  [unwired: 3 out]
                    n291 = Read from Binary File(5:sgl 0.0, 9:T9."little-endian" ("byte order (0:big-endian, network order)"), 10:-1 ("count (1)"), 11:w701) -> (0:w699:errorcluster, 2:w684:sgl[], 3:w700:refnum<file>)  [unwired: 1 in, 2 out]
                    n292 = Close File(refnum=w700, error in=w699) -> (error out=w695:errorcluster)  [unwired: 1 out]
                    n293 = local read "Series_flota"() -> (w690:string[])
                    n294 = call "Puntos medio de pulso.vi"("DI Inductivo"=w684) -> ("Puntos"=w710:sgl[], "Número de ejes"=w669:i32)  [unwired: 1 in]
                    n295 = Array Size(array=w684) -> (size(s)=w689:i32)
                    n296 = call "Distancias_ejes_convoy.vi"("Series_flota1"=w682, "Ejes_UT"=w672, "Puntos medios de las ventanas"=w693, "Series_flota"=w690) -> ("Distancias_entre_ejes_convoy"=w692:dbl[])  [unwired: 1 in]
                    n297 = Subtract(x=w689, y=3 ("length")) -> (x-y=w687:i32)
                    n298 = Delete From Array(array=w684, length=3, index=w687) -> (array with subset deleted=w685:sgl[])  [unwired: 1 out]
                    n299 = Decrement(x=w669) -> (x-1=w709:i32)
                    n300 = local read "Tiempo de paso (s)"() -> (w708:dbl)
                    n301 = local read "TAGs"() -> (w677:string[])
                    n302 = local read "it-LR6"() -> (w674:i32)
                    n303 = local read "it-read-LR6"() -> (w675:i32[])
                    n304 = local read "TAGs LR6"() -> (w676:string[])
                    n305 = local read "Plataformas?"() -> (w673:bool)
                    n306 = call "Calculo_Velocidad.vi"("Tiempo de paso (s)"=w708, "Ejes"=w709, "Puntos iniciales de las ventanas"=w692) -> ("V (m/s)"=→"V (m/s)":dbl, "Longitud de la unidad"=→"Longitud de la unidad":dbl)
                    n307 = call "TAGs_AURAwheel.vi"("Nº Ejes"=w672, "TAGs"=w677, "Ejes_convoy"=w671, "it-LR6"=w674, "TAGs LR6"=w676, "it-read-LR6"=w675, "Plataformas?"=w673) -> ("TAGS_AURA"=→"TAGs_AURAwheel":string[][])  [unwired: 1 in]
                    n308 = call "Comprobación Señal digital (SubVI).vi"("Inductivo"=w685) -> ("Señal digital?"=w680:bool)
                    n309 = Get Volume Info(11:path "c:/" ("path")) -> (1:→"Disco Duro Disponible (bytes)":i64)  [unwired: 1 in, 5 out]
                    n310 = Equal?(x=w669, y=w669) -> (x = y?=w678:bool)
                    n311 = And(x=w678, y=w680) -> (x .and. y?=w679:bool)
                    "Número de ejes detectados" <- 3 ("Número de ejes detectados")
                    "Nº Ejes" <- i32[] [3, 3] ("Nº Ejes")
                  }
                }
                n312 = case shown="True" w658 {
                  tunnel: w659 -> [w731 w761]
                  tunnel: [w731 w760] -> w666
                  tunnel: w665 -> [_ w765]
                  tunnel: w664 -> [_ w763]
                  tunnel: w657 -> [_ w764]
                  tunnel: w656 -> [w729 _]
                  frame False {
                    n313 = local read "Nombre de archivo"() -> (w730:path[])
                    n314 = for {
                      tunnel: w730 -> [w733] mode=indexing
                      tunnel: w729 -> [w732]
                      n315 = flat-sequence {
                        tunnel: w733 -> [w742]
                        tunnel: [w742] -> w736
                        tunnel: [w741] -> w735
                        tunnel: w732 -> [w740]
                        tunnel: w736 -> [w749]
                        tunnel: [w748] -> w734
                        tunnel: w735 -> [w748]
                        tunnel: w734 -> [w751]
                        frame #0 {
                          w741 = path "c:/Est_Adq.csv" ("file path (use dialog)")
                          n316 = Path To String(path=w742) -> (string=w744:string)
                          n317 = Select(t="Nº Ejes detectados WS diferente a Nº Ejes TAGs" ("delimiter (\\t)"), s=w740, f="La señal del inductivo no es digital" ("delimiter (\\t)")) -> (s? t:f=w737:string)
                          n318 = Build Array(w744, w737) -> (w743:string[])
                          n319 = call-poly <vilib>:"Write To Spreadsheet File.vi"("delimiter (\\t)"=";" ("delimiter (\\t)"), "transpose? (no:F)"=FALSE, "append to file? (new file:F)"=TRUE, "1D data"=w743, "file path (dialog if empty)"=w741) -> ()  [unwired: 3 in, 1 out]
                        }
                        frame #1 {
                          n320 = disable-structure shown="Disabled" {
                            disable-tunnel: w749 -> [w750 _]
                            frame Disabled {
                              n321 = Delete(path (use dialog)=w750) -> ()  [unwired: 1 in, 6 out]
                            }
                            frame Enabled {
                            }
                          }
                        }
                        frame #2 {
                          n322 = File/Directory Info(path=w751) -> (size=w754:i64)  [unwired: 1 in, 6 out]
                          n323 = Greater?(x=w754, y=i64 1000000) -> (0:w752:bool)
                          n324 = case shown="True" w752 {
                            tunnel: w751 -> [_ w755]
                            frame False {
                            }
                            frame True {
                              n325 = Delete(path (use dialog)=w755) -> ()  [unwired: 4 in, 3 out]
                            }
                          }
                        }
                      }
                    }
                  }
                  frame True {
                    n326 = flat-sequence {
                      tunnel: w765 -> [w831]
                      tunnel: w764 -> [w827]
                      tunnel: w763 -> [w832]
                      tunnel: [w825] -> w762
                      frame #0 {
                        # "Entrada:\n- dt RMS\n- Paths\n- Param_acelerometros (sensivity)\n- Parm_filtro\n- Puntos ventana\n- error\n- Frecuencia\n- Velocidad ejes\n- Punto medio paso rueda (p)"
                        # "SALIDA \n\nMáximos por rueda inductivo"
                        # "ENTRADA \nNúmero de ejes\nDistancia de acelerómetros\nDistancias del centro de las ruedas\nPuntos medios de las ruedas (INDUCTIVO)\nFrecuencia\ndt RMS\nDistancias generales\nAceleraciones"
                        # "8 acelerómetros"
                        # "Velocidad"
                        n327 = local read "Frecuencia de muestreo (Hz)"() -> (w830:dbl)
                        n328 = local read "Distancia de acelerómetros"() -> (w833:dbl[])
                        n329 = local read "Parámetros acelerómetros"() -> (w824:dbl[])
                        n330 = local read "Número de ejes detectados"() -> (w823:i32)
                        n331 = local read "Distancias generales"() -> (w828:dbl[])
                        n332 = local read "dt RMS"() -> (w829:dbl)
                        n333 = call "Procesado_aRMS_Zar.vi"("Número de ejes"=w823, "Distancias generales (m)"=w828, "array"=w827, "Parámetros acelerómetros 2"=w833, "Distancia de acelerómetros"=w824, "Frecuencia de muestreo"=w830, "dt RMS 2"=w829, "Distancias centrales de las ruedas\n               configuración (m)"=w832, "Puntos"=w831) -> ("Max RMS Ruedas"=w826:dbl[][])
                        n334 = Transpose 2D Array(2D array=w826) -> (transposed array=w825:dbl[][])
                        "Max RMS Ruedas" <- w825
                      }
                    }
                    n335 = disable-structure shown="Disabled" {
                      disable-tunnel: [w821 TRUE ("Use Aura?")] -> w759
                      frame Disabled {
                        n336 = local read "Use Aura?"() -> (w821:bool)
                      }
                      frame Enabled {
                      }
                    }
                    n337 = local read "TAGs_AURAwheel"() -> (w757:string[][])
                    n338 = local read "Nº Ejes"() -> (w756:i32[])
                    n339 = for {
                      tunnel: w759 -> [w770]
                      tunnel: [w769] -> w758 mode=indexing
                      tunnel: w757 -> [w768] mode=indexing
                      shift-right: [w767] -> _
                      shift-left: w762 -> [w771]
                      tunnel: w756 -> [w766] mode=indexing
                      # "dev.api.aurawheel.com"
                      n340 = case shown="True" w770 {
                        tunnel: w771 -> [w772 w778]
                        tunnel: [errorcluster {"status"=FALSE, "code"=0, "source"=""} ("error out") w790] -> w769
                        tunnel: w768 -> [_ w779]
                        tunnel: [w772 w777] -> w767
                        tunnel: w766 -> [_ w775]
                        frame False {
                        }
                        frame True {
                          (unwired) "http://dev.api.aurawheel.com/services/wrd/upload"
                          (unwired) "tagMexFin"
                          (unwired) "tagMexInit"
                          (unwired) "tag2"
                          (unwired) "tag1"
                          w794 = cluster{"status":string} {"status"=""}
                          n341 = local read "TAGs"() -> (w785:string[])
                          n342 = local read "Parametros AuraWheel"() -> (w819:string[])
                          n343 = Delete From Array(array=w778, length=w775, index (row)=0) -> (deleted portion=w774:dbl[][], array with subset deleted=w777:dbl[][])  [unwired: 1 in]
                          n344 = Get Date/Time In Seconds() -> (seconds since 1Jan1904=w815:timestamp)
                          n345 = Delete From Array(array=w785, length=2, index=0) -> ()  [unwired: 2 out]
                          n346 = Format Date/Time String(time format string (%c)="%H:%M:%S%3u", seconds (now)=w815) -> (date/time string=w813:string)  [unwired: 1 in]
                          n347 = Get Date/Time In Seconds() -> (seconds since 1Jan1904=w789:timestamp)
                          n348 = Scan From String(format string="%d:%d:%f", input string=w813) -> (output 1=w810:i32, output 2=w809:i32, output 3=w807:dbl)  [unwired: 5 in, 3 out]
                          n349 = local read "Temperatura (ºC)"() -> (w787:dbl)
                          n350 = disable-structure shown="Enabled" {
                            disable-tunnel: [_ 60.0 ("p_sp")] -> w786
                            frame Disabled {
                              n351 = local read "V (m/s)"() -> ()  [unwired: 1 out]
                            }
                            frame Enabled {
                            }
                          }
                          n352 = Multiply(x=w807, y=1000.0) -> (x*y=w803:dbl)
                          n353 = call "Time_to_ms.vi"("seconds since 1Jan1904"=w789) -> ("Numeric"=w788:dbl)  [unwired: 1 in]
                          n354 = Multiply(x=w809, y=60000) -> (x*y=w804:i32)
                          n355 = Multiply(x=3600000, y=w810) -> (x*y=w805:i32)
                          n356 = Index Array(array=w819) -> ()  [unwired: 3 in, 3 out]
                          n357 = call "aw_WRDCluster_8acel.vi"("Array TAGs"=w779, "Max RMS Ruedas"=w774, "TimeStamp"=w788, "p_sp"=w786, "p_tp"=w787) -> ("JSON cluster"=w816:T11)  [unwired: 1 in]
                          n358 = Compound Arithmetic op=ADD(w805, w804, w803) -> (w802:dbl)
                          n359 = To Variant(anything=w816) -> (Variant=w799:variant)
                          n360 = To Unsigned Long Integer(number=w802) -> (unsigned 32bit integer=w801:u32)
                          n361 = call "gjson_Create.vi"("JSON Object in"=w799) -> ("error out"=w797:errorcluster, "JSON String Out"=w798:string)  [unwired: 9 in]
                          n362 = Number To Decimal String(number=w801) -> (decimal integer string=w800:string)  [unwired: 1 in]
                          n363 = To Variant(anything=w794) -> (Variant=w793:variant)
                          n364 = call "aw_SendData.vi"("pwd"="wrd", "x-nem-datetime"=w800, "User"="User", "error in"=w797, "JSON Object"=w798, "URL"="http://api.aurawheel.dev/services/wrd/upload") -> ("error out"=w795:errorcluster, "Response JSON"=w796:string, "Response headers"=→"Response headers":string)  [unwired: 3 in]
                          n365 = call "gjson_Parse.vi"("error in"=w795, "JSON String In"=w796, "JSON Cluster"=w793) -> ("error out"=w791:errorcluster, "JSON Cluster Out"=w792:variant)  [unwired: 7 in]
                          n366 = Variant To Data(error in=w791, type=w794, Variant=w792) -> (data=→"data":cluster{"status":string}, error out=w790:errorcluster)
                          "error AURA" <- w790
                        }
                      }
                    }
                    n367 = Merge Errors(w758, w761) -> (w760:errorcluster)
                  }
                }
              }
              frame #1 {
                n368 = local read "TAGS leidos"() -> (w837:path)
                n369 = local read "Nombre de archivo"() -> (w834:path[])
                n370 = File/Directory Info(path=w837) -> (size=w840:i64)  [unwired: 1 in, 6 out]
                n371 = local read "Path TEST"() -> (w836:path)
                n372 = disable-structure shown="Disabled" {
                  frame Disabled {
                    n373 = call "Borrar_carpeta.vi"("Nº Archivos Max"=1000, "Path Carpeta"=path "c:/Trenes") -> ()  [unwired: 1 in]
                  }
                  frame Enabled {
                  }
                }
                n374 = Greater?(x=w840, y=i64 1000000) -> (0:w838:bool)
                n375 = case shown="True" w838 {
                  tunnel: w837 -> [_ w846]
                  frame False {
                  }
                  frame True {
                    n376 = Delete(path (use dialog)=w846) -> ()  [unwired: 4 in, 3 out]
                  }
                }
                n377 = call "Borrar_carpeta.vi"("Nº Archivos Max"=i64 250 ("y"), "Path Carpeta"=w836) -> ()  [unwired: 1 in]
                n378 = call "Retrieve_memory_3_folders.vi"() -> ()  [unwired: 12 in]
                n379 = call "Comprimir_a_1_archivo.vi"("Acel_paths"=w834) -> ()  [unwired: 1 out]
              }
            }
            n380 = disable-structure shown="Disabled" {
              disable-tunnel: [w655 _] -> w629
              frame Disabled {
                n381 = local read "IP synchr"() -> (w654:string)
                n382 = call "Synchronization.vi"("Time Server\nIP Address"=w654) -> ("error out"=w655:errorcluster)
              }
              frame Enabled {
              }
            }
            n383 = call <vilib>:"Watchdog Clear.vi"("error in (no error)"=w648, "watchdogID in"=w647) -> ("error out"=w646:errorcluster)  [unwired: 5 out]
            n384 = local read "RFID_Error"() -> (w634:errorcluster)
            n385 = Merge Errors(w644, w646) -> (w635:errorcluster)
            n386 = Merge Errors(w630, w629, w634, w635) -> (w645:errorcluster)
            n387 = Unbundle By Name(w645) -> ("status"=w639:bool)
            n388 = Select(t="Descarga datos", s=FALSE, f="Espera") -> (s? t:f=w641:string)
            n389 = Select(t="TEST", s=w639, f=w641) -> (s? t:f=w638:string)
          }
          frame "TEST" {
            n390 = local read "expiration actions"() -> (w848:T1)
            n391 = call <vilib>:"Watchdog Configure.vi"("expiration actions"=w848, "timeout (1 sec)"=200.0) -> ("error out"=w851:errorcluster, "watchdogID"=w852:u64)  [unwired: 1 in, 3 out]
            n392 = flat-sequence {
              tunnel: [w863] -> w858
              tunnel: w857 -> [w883]
              tunnel: w855 -> [w882]
              tunnel: [w881] -> w854
              tunnel: w852 -> [w872]
              tunnel: w851 -> [w871]
              tunnel: [w870] -> w850
              tunnel: [w869] -> w849
              tunnel: [w859] -> w847
              frame #0 {
                n393 = call <vilib>:"Watchdog Whack.vi"("error in (no error)"=w871, "reset watchdog after expire? (F)"=TRUE, "watchdogID in"=w872) -> ("error out"=w869:errorcluster, "watchdogID out"=w870:u64)  [unwired: 3 out]
                n394 = Get Date/Time In Seconds() -> (seconds since 1Jan1904=w875:timestamp)
                n395 = local read "Ultimo TEST"() -> (w876:timestamp)
                n396 = To Double Precision Float(number=w875) -> (double precision float=w877:dbl)
                n397 = Subtract(x=w877, y=3600.0) -> (x-y=w879:dbl)
                n398 = To Time Stamp(1:w879) -> (0:w880:timestamp)
                n399 = In Range and Coerce(upper limit=w875, x=w876, lower limit=w880) -> (In Range?=w874:bool)  [unwired: 1 out]
                n400 = case shown="False" w874 {
                  tunnel: w883 -> [w913 _]
                  tunnel: w882 -> [w888 w919]
                  tunnel: [w898 errorcluster {"status"=FALSE, "code"=0, "source"=""} ("error out")] -> w881
                  tunnel: [w888 w919] -> w859
                  frame False {
                    n401 = local read "Obstruido?"() -> (w890:bool)
                    n402 = case shown="True" w890 {
                      selector: w890 -> [_ w915]
                      tunnel: ["\r" w916] -> w887
                      frame False {
                      }
                      frame True {
                        n403 = call "ErrorObstruccion.vi"("Buffer Overflow"=w915) -> ("error out"=w918:errorcluster)
                        n404 = call "Error.vi"("Error con..."="Warning:", "error comunicacion 2"=w918) -> ("String"=w916:string)
                      }
                    }
                    n405 = local read "Aviso no detección"() -> (w896:string)
                    n406 = local read "Aviso temperatura"() -> (w895:string)
                    n407 = local read "RFID_Error"() -> (w892:errorcluster)
                    n408 = local read "RFID_LR6_Error"() -> (w885:errorcluster)
                    n409 = local read "DC OK"() -> (w894:string)
                    n410 = local read "Fallo sensores"() -> (w889:string)
                    n411 = call "Cabecera.vi"() -> ("String"=w911:string)
                    n412 = call "Adquisicion.vi"("Aviso no detección"=w896) -> ("String"=w910:string)
                    n413 = call "Temperatura.vi"("Aviso temperatura"=w895) -> ("String"=w909:string)
                    n414 = call "Fuente.vi"("DC OK"=w894) -> ("String"=w908:string)
                    n415 = call "FPGA.vi"("error out"=w888) -> ("String"=w907:string)
                    n416 = call "Escritura.vi"("error out"=w913) -> ("String"=w906:string)
                    n417 = call "Error.vi"("Error con..."="Error con el lecto RFID NEM", "error comunicacion 2"=w892) -> ("String"=w891:string)
                    n418 = call "Error.vi"("Error con..."="Error con el lecto RFID LR6-HD", "error comunicacion 2"=w885) -> ("String"=w884:string)
                    n419 = Concatenate Strings(w911, w910, w909, w908, w907, w906, w889, w891, w884, w887) -> (w912:string)
                    n420 = call "STRINGhorafechA(SubVI).vi"() -> ("STRINGhora_fecha"=w905:string)
                    n421 = Concatenate Strings(w905, ".txt" ("string")) -> (w901:string)
                    n422 = Get Date/Time In Seconds() -> (seconds since 1Jan1904=→"Ultimo TEST":timestamp)
                    n423 = Build Array("c", "TEST" ("element"), w901) -> (w903:string[])
                    n424 = Array of Strings to Path(0:w903) -> (2:w899:path)  [unwired: 1 out]
                    n425 = Write to Text File(file (use dialog)=w899, text=w912) -> (error out=w898:errorcluster)  [unwired: 1 in, 3 out]
                  }
                  frame True {
                  }
                }
                n426 = local read "Fallo fotocelula"() -> (w862:bool)
                n427 = Unbundle By Name(w859) -> ("status"=w860:bool)
                n428 = local read "T fuera rango"() -> (w868:bool)
                n429 = Compound Arithmetic op=OR(w860, w862) -> (w861:bool)
                n430 = local write "Reset del controlador"(w861) -> ()
                n431 = Select(t="Escape", s=w868, f="Espera") -> (s? t:f=w865:string)
                n432 = Select(t="Configuracion", s=w861, f=w865) -> (s? t:f=w863:string)
              }
            }
            n433 = call <vilib>:"Watchdog Clear.vi"("error in (no error)"=w849, "watchdogID in"=w850) -> ()  [unwired: 6 out]
          }
          frame "Escape" {
            n434 = while {
              tunnel: w924 -> [w940]
              tunnel: [w939] -> w925
              shift-right: [w938] -> w922
              shift-left: w921 -> [w927]
              stop <- w930 stop-if-true
              # "Espera hasta que el detector de\npresencia se desactive"
              n435 = Wait (ms)(milliseconds to wait=u32 3000) -> ()  [unwired: 1 out]
              n436 = xnode "Read/Write Control"("FPGA VI Reference In"=w940, "error in"=w927) -> ("FPGA VI Reference Out"=w939:refnum<k20>, "error out"=w938:errorcluster, "Detector de presencia"=w936:bool, "Chassis Temperature"=w931:i16)
              n437 = Divide(x=w931, y=4.0) -> (x/y=w932:dbl)
              n438 = In Range and Coerce(upper limit=55.0, x=w932, lower limit=0.0) -> (In Range?=w928:bool)  [unwired: 1 out]
              n439 = Not(x=w936) -> (.not. x?=w929:bool)
              n440 = And(x=w929, y=w928) -> (x .and. y?=w930:bool)
            }
          }
        }
        "Estado" <- w66
        "error manipulacion archivos" <- w68
        n441 = local read "Parar la aplicación"() -> (w65:bool)
      }
      n442 = xnode "Close FPGA VI Reference"("FPGA VI Reference In"=w58, "error in"=w57) -> ("error out"=→"error FPGA":errorcluster)
    }
    frame #3 {
      n443 = local read "RFID_ID"() -> (w943:refnum<k5>)
      n444 = call "LH6HD.vi"("Action"=enum16{"Init", "Start", "Read", "Stop", "Exit"}."Stop") -> ("error out"=→"RFID_LR6_Error":errorcluster)  [unwired: 9 in, 1 out]
      n445 = TCP Close Connection(connection ID=w943) -> (error out=→"RFID_Error":errorcluster)  [unwired: 1 in, 2 out]
    }
  }
